vi "Main.vi"() -> ()   [LabVIEW 2016]
panel:
  in  "stop":bool
  in  "Tab Control":enum32{"Navigation", "Interface", "About"}(tab)
  in  "Reference Auto Update 3":bool=TRUE caption="Auto Update"
  out "move out":bool=TRUE caption="Move"
  in  "Positioner 2":u16(ring)=15 caption="Positioner" items=["ECGp5050", "ECGt5050", "ECR3030", "ECR4040", "ECR5050", "ECSx3030", "ECSx3040", "ECSx3050", "ECSx3060", "ECSx3070", "ECSx3080", "ECSx5050", "ECSxy5050", "ECSz3030", "ECSz5050", "EOP1", "EOP2"]
  out "in target range3":bool
  in  "auto Reset 1":bool=TRUE caption="Auto Reset"
  in  "Target Range 3":u32 caption="Target Range"
  in  "Reset Error 2":bool
  in  "Reset Error 3":bool
  out "Error 3":bool caption="Error"
  out "Error Message 3":string
  out "actor type 2":u16(ring) caption="Status" items=["linear positioner"=0, "rotator"=1, "goniometer"=2, "< error >"=9]
  out "actor type":u16(ring) caption="Status" items=["linear positioner"=0, "rotator"=1, "goniometer"=2, "< error >"=9]
  out "EotLeftDetected3":bool caption="Status Eot BWD"
  out "EotrightDetected3":bool caption="Status Eot FWD"
  in  "EoT 3":bool=TRUE caption="Stop on EoT"
  out "EotLeftDetected2":bool caption="Status Eot BWD"
  out "EotrightDetected2":bool caption="Status Eot FWD"
  in  "EoT 2":bool=TRUE caption="Stop on EoT"
  in  "Move 3":bool
  out "MoveSignal 3":bool caption="Positioner Connected/Moving"
  out "MoveSignal":bool caption="Positioner Connected/Moving"
  out "ReferenceSignal":bool=TRUE
  in  "Axis 3":bool caption="Closed Loop Funktions"
  in  "Axis 2":bool caption="Closed Loop Funktions"
  in  "Target Position 3":i32 caption="Target Position [µm]"
  in  "Target Position 1":i32 caption="Target position [µm]"
  in  "Number of steps 3":i32=1 caption="Number of Steps"
  in  "Number of steps 2":i32=1 caption="Number of Steps"
  in  "Output 2":bool caption="Axis 2"
  in  "Move 2":bool
  in  "Move":bool
  out "ReferenceSignal 3":bool
  out "Reference 3":dbl caption="Reference position [nm]" format="%#_6f"
  in  "Output":bool=TRUE caption="Axis 1"
  out "Output Satus 3":bool caption="Output Status"
  in  "Reference Auto Update 2":bool=TRUE caption="Auto Update"
  out "Error Message":string
  out "Error":bool
  in  "Output 3":bool caption="Axis 3"
  in  "auto Reset 3":bool=TRUE caption="Auto Reset"
  out "Output Status 1":bool=TRUE caption="Output Status"
  out "Position 3":dbl caption="Position [nm]" format="%#_6f"
  out "Output Status 2":bool caption="Output Status"
  in  "amplitude [V] 3":dbl=45.001 caption="Amplitude [V]" format="%#.3f"
  in  "frequency [Hz] 3":dbl=997.363 caption="Frequency [Hz]" format="%#.3f"
  out "Error 2":bool caption="Error"
  out "actor type 3":u16(ring) caption="Status" items=["linear positioner"=0, "rotator"=1, "goniometer"=2, "< error >"=9]
  out "Error Message 2":string
  out "Connected 3":bool caption="Connected"
  in  "Single Step Left 3":bool caption="Open Loop Funktions"
  in  "Positioner 3":u16(ring)=15 caption="Positioner" items=["ECGp5050", "ECGt5050", "ECR3030", "ECR4040", "ECR5050", "ECSx3030", "ECSx3040", "ECSx3050", "ECSx3060", "ECSx3070", "ECSx3080", "ECSx5050", "ECSxy5050", "ECSz3030", "ECSz5050", "EOP1", "EOP2"]
  in  "Endless Left 3":bool caption="Continuous Backward"
  in  "Continuous Forward":bool
  in  "Single Step Right 3":bool caption="Step(s)"
  in  "Fixed DC 3":i32 caption="DC Level [mV]"
  out "move out 3":bool=TRUE caption="Move"
  out "Position 2":dbl caption="Position [nm]" format="%#_6f"
  in  "amplitude [V] 2":dbl=45.001 caption="Amplitude [V]" format="%#.3f"
  in  "Amplitude [V]":dbl=45.001 format="%#.3f"
  in  "frequency [Hz] 2":dbl=997.363 caption="Frequency [Hz]" format="%#.3f"
  in  "Frequency [Hz]":dbl=1998.531 format="%#.3f"
  out "Connected 2":bool caption="Connected"
  in  "Single Step Left":bool caption="Open Loop Funktions"
  in  "Single Step Left 2":bool caption="Open Loop Funktions"
  in  "Single Step Right 2":bool caption="Step(s)"
  in  "Number of steps 1":i32=1 caption="Number of Steps"
  out "ReferenceSignal 2":bool
  in  "Single Step Right":bool caption="Step(s)"
  in  "Endless Left":bool caption="Continuous Backward"
  in  "Continuous Forward":bool
  in  "Endless Left 2":bool caption="Continuous Backward"
  out "EotLeftDetected1":bool caption="Status Eot BWD"
  out "EotrightDetected1":bool caption="Status Eot FWD"
  in  "EoT 1":bool caption="Stop on EoT"
  in  "Target position 2":i32 caption="Target Position [µm]"
  out "in target range2":bool
  in  "Continuous Forward":bool
  out "Reference 2":dbl caption="Reference position [nm]" format="%#_6f"
  in  "Fixed DC 2":i32 caption="DC Level [mV]"
  out "MoveSignal 2":bool caption="Positioner Connected/Moving"
  out "in target range1":bool
  in  "Target Range 2":u32 caption="Target Range [nm]"
  in  "Target Range 1":u32 caption="Target Range"
  out "Reference":dbl=-7597148.0 caption="Reference position [nm]" format="%#_6f"
  in  "auto Reset 2":bool=TRUE caption="Auto Reset"
  out "Position":dbl=14701.126 caption="Position [nm]" format="%#_6f"
  in  "Axis 1":bool caption="Closed Loop Funktions"
  in  "Fixed DC 1":i32 caption="DC Level [mV]"
  out "move out 2":bool=TRUE caption="Move"
  in  "Reset Error":bool
  out "Connected":bool=TRUE
  in  "Positioner":u16(ring)=15 items=["ECGp5050", "ECGt5050", "ECR3030", "ECR4040", "ECR5050", "ECSx3030", "ECSx3040", "ECSx3050", "ECSx3060", "ECSx3070", "ECSx3080", "ECSx5050", "ECSxy5050", "ECSz3030", "ECSz5050", "EOP1", "EOP2"]
  in  "Reference Auto Update 1":bool=TRUE caption="Auto Update"
  out "Error 4":bool caption="Error"
  out "Error Message 4":string
  in  "Mode Input 1":u16(ring) caption="Mode" items=["Trigger (LVDS)"=11, "Trigger (LVTTL)"=10, "Stepper (LVDS)"=9, "Stepper (LVTTL)"=8, "AquadB (LVDS)"=1, "AquadB (LVTTL)"=0, "OFF"=15]
  in  "Loop Mode 1":u16(ring) caption="Loop mode" items=["closed-loop"=1, "open-loop"=0]
  in  "Steps per pulse 1":i32 caption="Steps per pulse [Steps]"
  in  "Change per pulse 1":i32 caption="Change per pulse [u°/nm]"
  out "RT in move Signal 1":bool=TRUE caption="move"
  in  "RT in move 1":bool=TRUE caption="Move"
  in  "AquadB in res 1":i32 caption="AquadB Resolution [nm]"
  in  "AquadB out 1":bool caption="AquadB enable"
  in  "AqaudB clock 1":i32 caption="AquadB Clock [ns]"
  in  "AquadB Resolution 1":i32 caption="AquadB Resolution [nm]"
  in  "Reset Error 4":bool
  out "Error 5":bool caption="Error"
  out "Error Message 5":string
  in  "Mode Input 2":u16(ring) caption="Mode" items=["Trigger (LVDS)"=11, "Trigger (LVTTL)"=10, "Stepper (LVDS)"=9, "Stepper (LVTTL)"=8, "AquadB (LVDS)"=1, "AquadB (LVTTL)"=0, "OFF"=15]
  in  "Loop Mode 2":u16(ring) caption="Loop mode" items=["closed-loop"=1, "open-loop"=0]
  in  "Steps per pulse 2":i32 caption="Steps per pulse [Steps]"
  in  "Change per pulse 2":i32 caption="Change per pulse  [u°/nm]"
  out "RT in move Signal 2":bool=TRUE caption="move"
  in  "RT in move 2":bool=TRUE caption="Move"
  in  "AquadB in res 2":i32 caption="AquadB Resolution [nm]"
  in  "AquadB out 2":bool caption="AquadB enable"
  in  "AqaudB clock 2":i32 caption="AquadB Clock [ns]"
  in  "AquadB Resolution 2":i32 caption="AquadB Resolution [nm]"
  in  "Reset Error 5":bool
  out "Error 6":bool caption="Error"
  out "Error Message 6":string
  in  "Mode Input 3":u16(ring) caption="Mode" items=["Trigger (LVDS)"=11, "Trigger (LVTTL)"=10, "Stepper (LVDS)"=9, "Stepper (LVTTL)"=8, "AquadB (LVDS)"=1, "AquadB (LVTTL)"=0, "OFF"=15]
  in  "Loop Mode 3":u16(ring) caption="Loop mode" items=["closed-loop"=1, "open-loop"=0]
  in  "Steps per pulse 3":i32 caption="Steps per pulse [Steps]"
  in  "Change per pulse 3":i32 caption="Change per pulse  [u°/nm]"
  out "RT in move Signal 3":bool=TRUE caption="move"
  in  "RT in move 3":bool=TRUE caption="Move"
  in  "AquadB in res 3":i32 caption="AquadB Resolution [nm]"
  in  "Output Mode":u16(ring) caption="Mode" items=["AquadB (LVTTL)", "AquadB (LVDS)"]
  in  "AquadB out 3":bool caption="AquadB enable"
  in  "AqaudB clock 3":i32 caption="AquadB Clock [ns]"
  in  "AquadB Resolution 3":i32 caption="AquadB Resolution [nm]"
  in  "Reset Error 6":bool
  in  "Reboot":bool
  in  "Factory Reset":bool
  in  "Reset Error 8":bool
  out "Error Message 7":string
  in  "Lock password":string
  in  "name":string="Test" caption="Device Name"
  in  "Access Password":string
  out "Error 7":bool caption="Error"
  out "locked":bool
  out "authorized":bool
  in  "Unlock":bool=TRUE
  out "Name":string caption="Device Name"
  out "Device type":string="AMC100/NUM"
  out "Sn":string caption="Serial Number"
  out "ip":string="192.168.1.1" caption="IP Adress"
  out "Firmware Version":string
  out "FPGA Version":string
  out "Mac Adress":string
  # "Real Time Input"
  # "Real Time Output"
  # "Global Parameters"
  # "Axis 1"
  # "Axis 1"
  # "Axis 2"
  # "Axis 2"
  # "Axis 3"
  # "Axis 3"
  # "Device Info"
  # "Device Access"
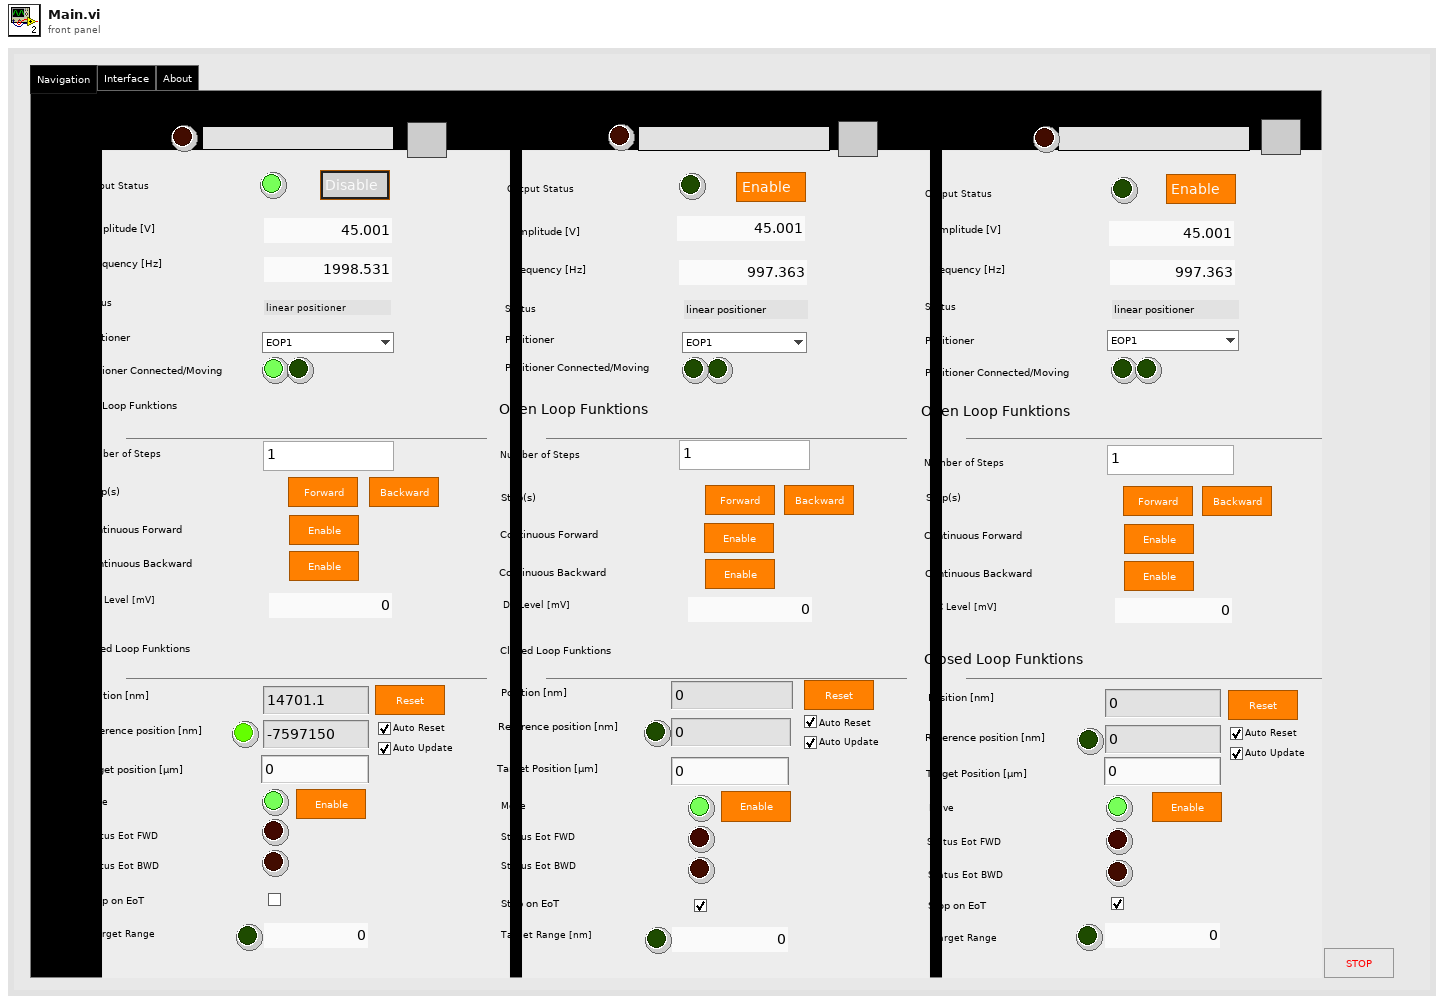
[diagram p1: front panel]
types:
  T1 = enum8{"Enabled", "Disabled", "Disabled and Grayed Out"}
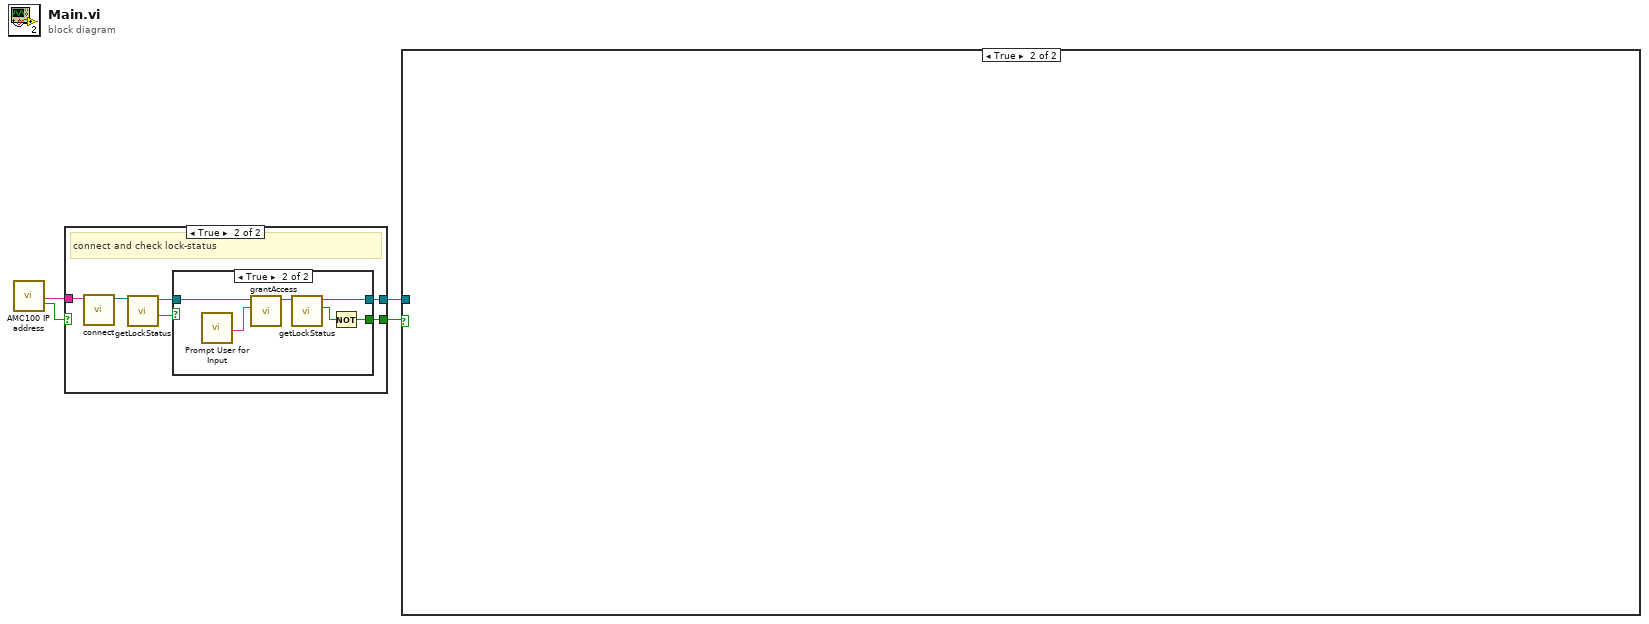
[diagram p0: block diagram]
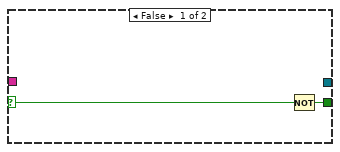
[diagram p2: hidden frame]
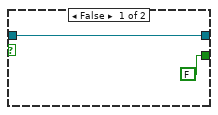
[diagram p3: hidden frame]
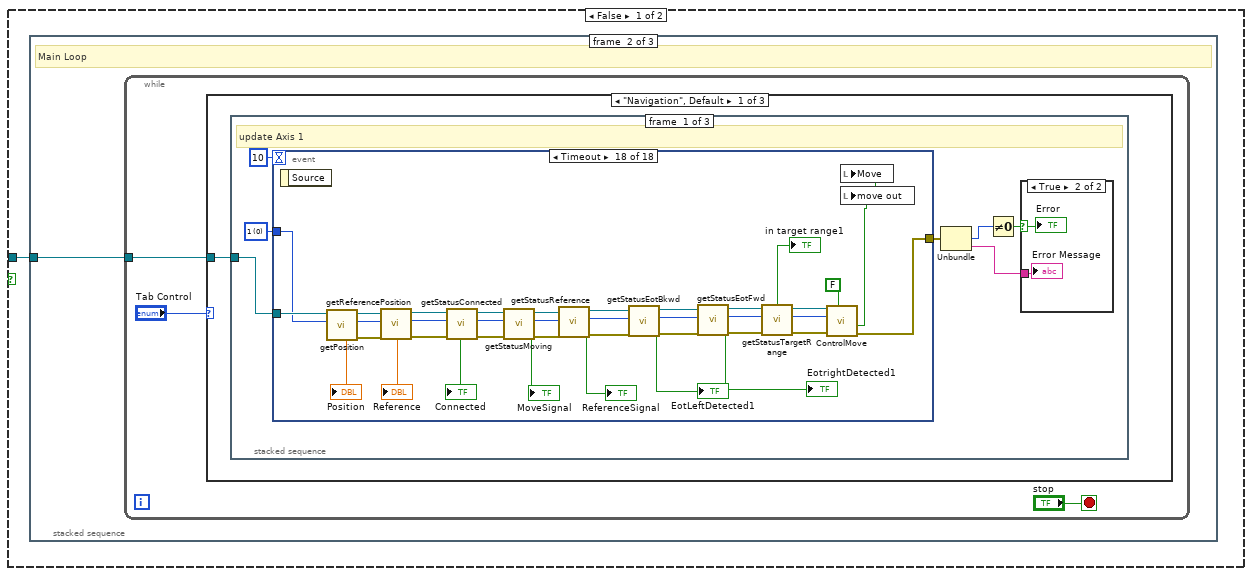
[diagram p4: hidden frame]
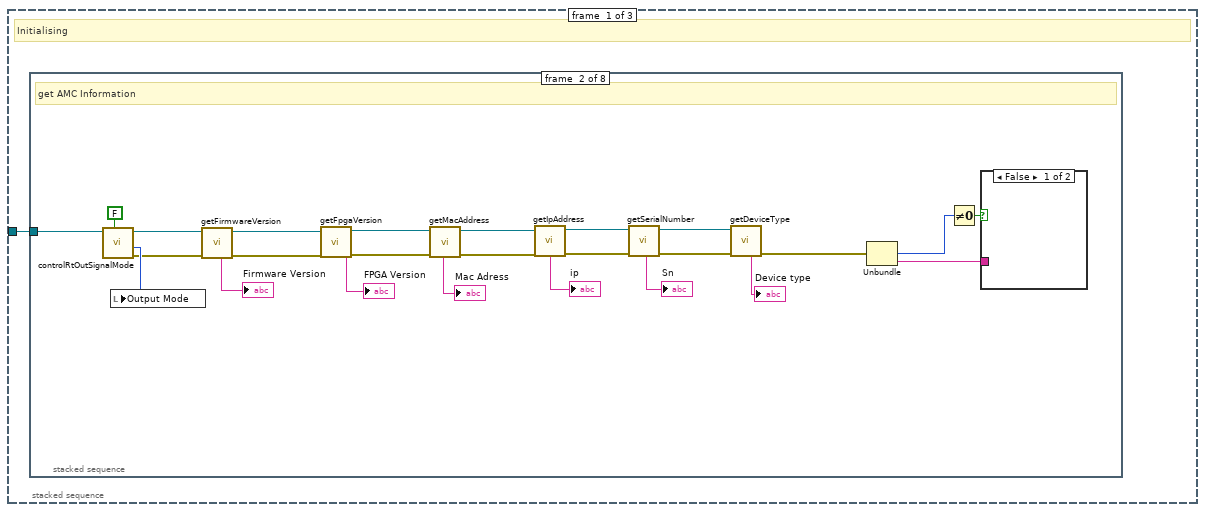
[diagram p5: hidden frame]
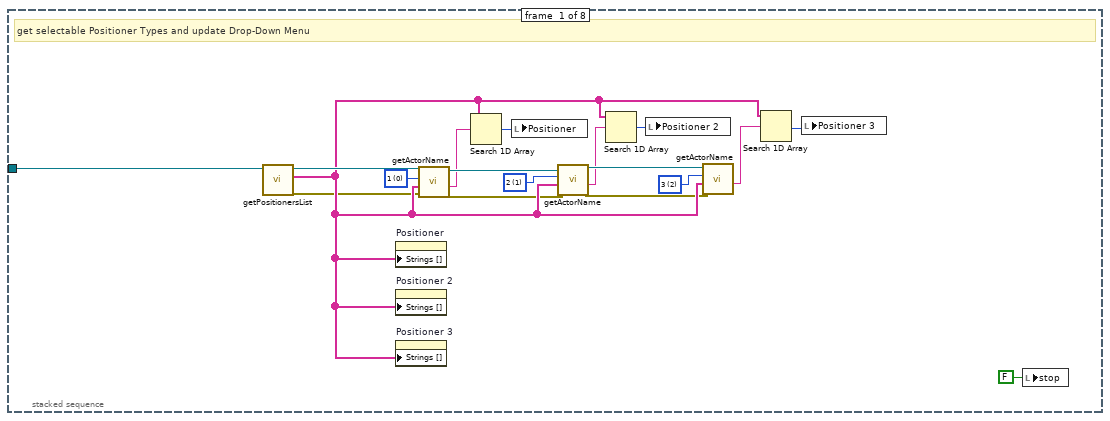
[diagram p6: hidden frame]
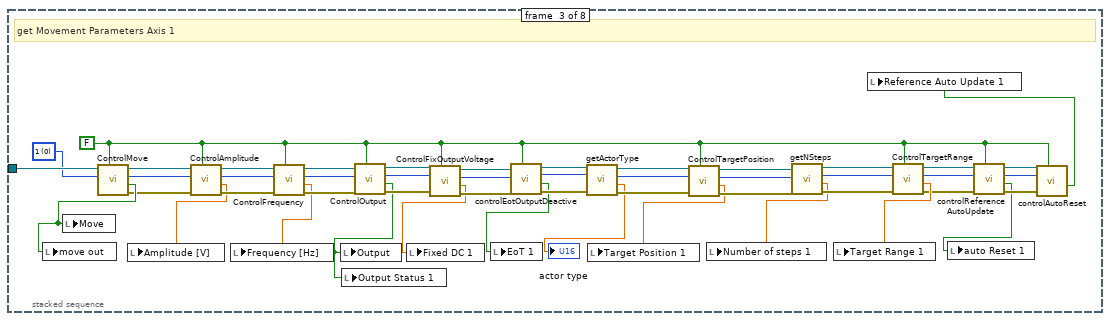
[diagram p8: hidden frame]
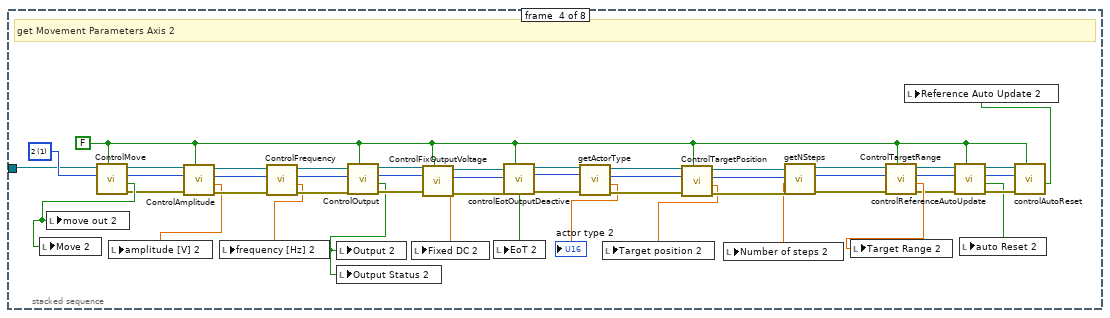
[diagram p9: hidden frame]
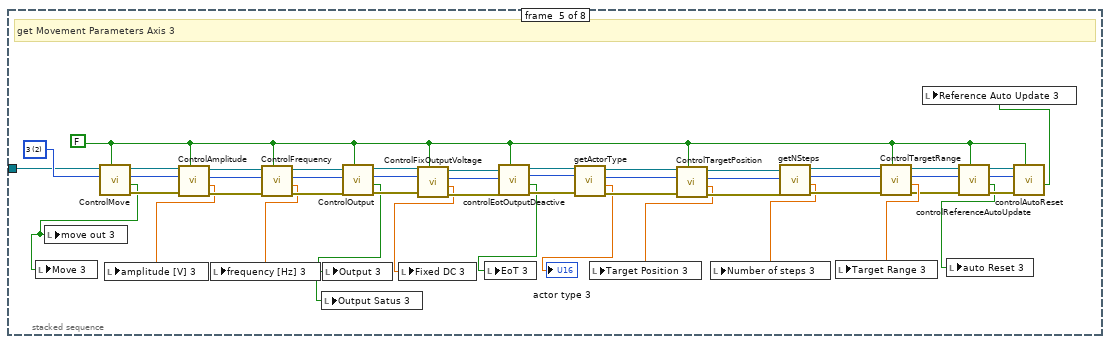
[diagram p10: hidden frame]
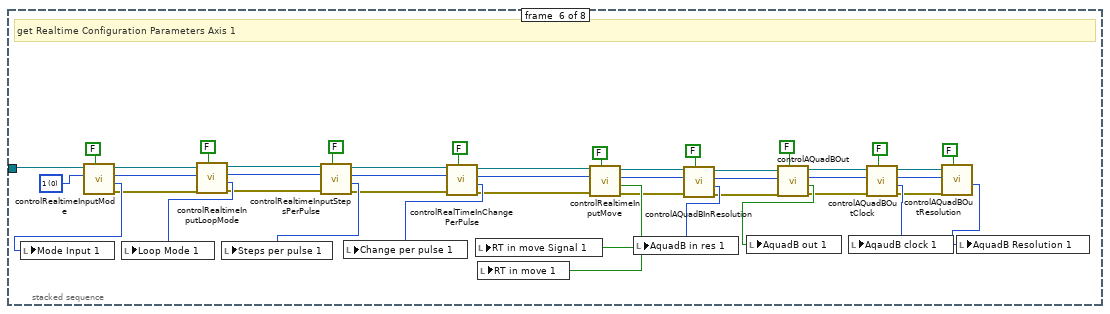
[diagram p11: hidden frame]
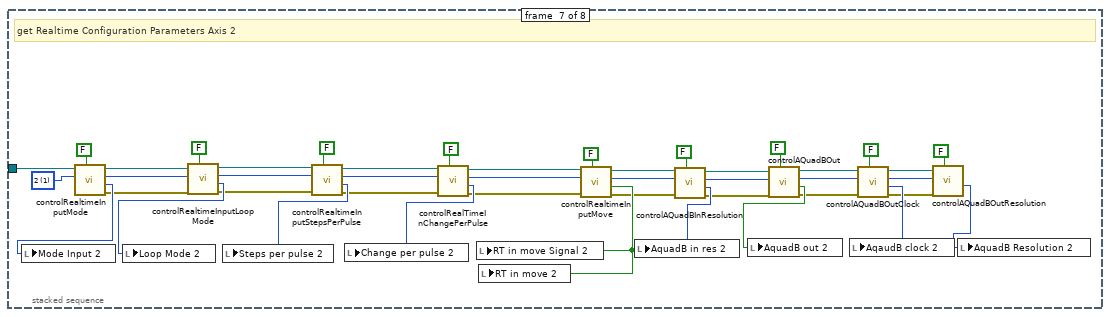
[diagram p12: hidden frame]
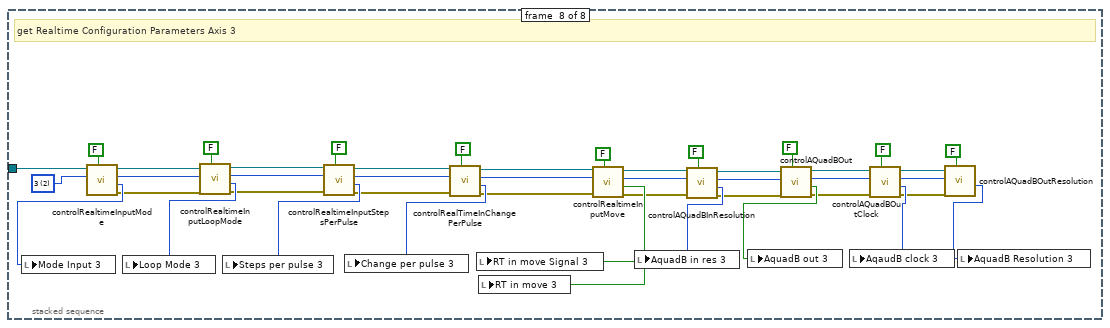
[diagram p13: hidden frame]
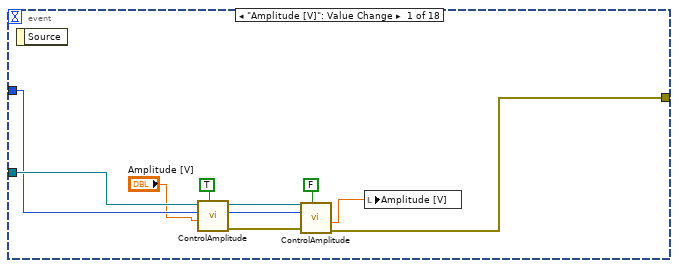
[diagram p15: hidden frame]
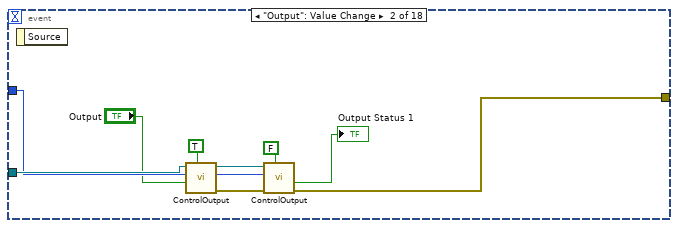
[diagram p16: hidden frame]
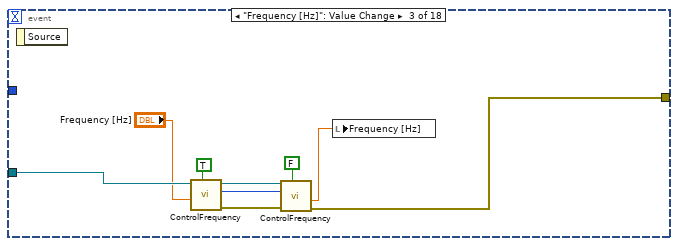
[diagram p17: hidden frame]
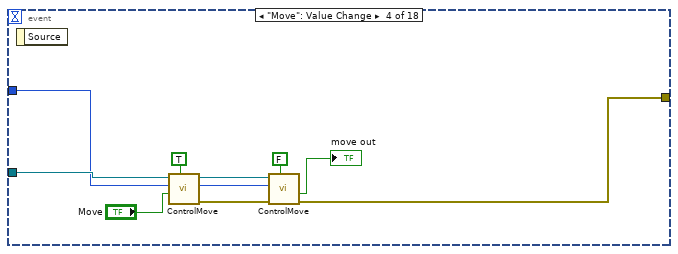
[diagram p18: hidden frame]
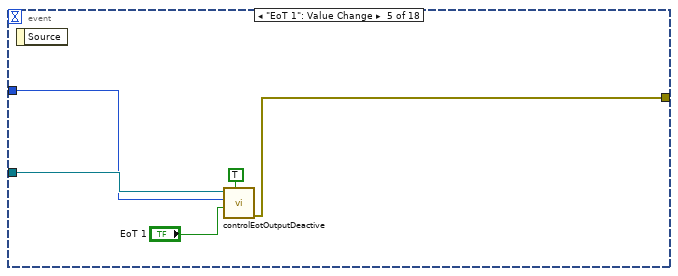
[diagram p19: hidden frame]
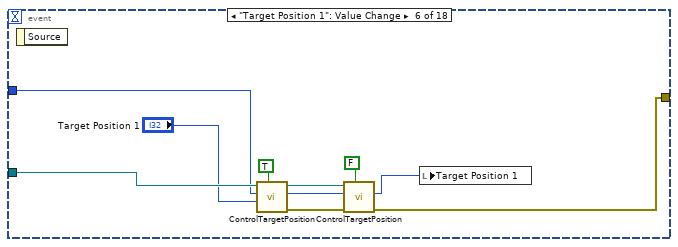
[diagram p20: hidden frame]
diagram:
  n1 = call "AMC100 IP address"() -> ("IP address"=w1:string, "OK"=w2:bool)  [unwired: 17 in, 1 out]
  n2 = case shown="True" w2 {
    selector: w2 -> [w5 _]
    tunnel: [w6 w12] -> w4
    tunnel: [_ w11] -> w3
    tunnel: w1 -> [_ w7]
    frame False {
      n3 = Not(x=w5) -> (.not. x?=w6:bool)
    }
    frame True {
      # "connect and check lock-status"
      n4 = call "connect.vi"("deviceAddress"=w7) -> ("connection ID"=w10:refnum<k5>)  [unwired: 5 in, 1 out]
      n5 = call "getLockStatus.vi"("connection ID in"=w10) -> ("locked"=w8:bool, "connection ID out"=w9:refnum<k5>)  [unwired: 7 in, 2 out]
      n6 = case shown="True" w8 {
        tunnel: w9 -> [w14 w20]
        tunnel: [w14 w17] -> w11
        tunnel: [FALSE w16] -> w12
        frame False {
        }
        frame True {
          n7 = call "Prompt User for Input"() -> ("password"=w19:string)  [unwired: 17 in, 2 out]
          n8 = call "grantAccess.vi"("password"=w19, "connection ID"=w20) -> ("connection ID"=w18:refnum<k5>)  [unwired: 8 in, 1 out]
          n9 = call "getLockStatus.vi"("connection ID in"=w18) -> ("authorized"=w15:bool, "connection ID out"=w17:refnum<k5>)  [unwired: 7 in, 2 out]
          n10 = Not(x=w15) -> (.not. x?=w16:bool)
        }
      }
    }
  }
  n11 = case shown="True" w4 {
    tunnel: w3 -> [w21 _]
    frame False {
      n12 = stacked-sequence {
        tunnel: w21 -> [w22 w342 w1332]
        frame #0 {
          # "Initialising"
          n13 = stacked-sequence {
            tunnel: w22 -> [w40 w44 w72 w120 w166 w253 w297 w341]
            frame #0 {
              w37 = u8 2 items=["1", "2", "3"] ("axis")
              w34 = u8 1 items=["1", "2", "3"] ("axis")
              w31 = u8 0 items=["1", "2", "3"] ("axis")
              # "get selectable Positioner Types and update Drop-Down Menu"
              n14 = call "getPositionersList.vi"("connection ID"=w40) -> ("error out"=w23:errorcluster, "Positioners List"=w26:string[], "connection ID"=w30:refnum<k5>)  [unwired: 8 in]
              n15 = property on="Positioner" class="Ring (strict)"("Strings []"=w26) -> ()  [unwired: 2 in, 2 out]
              n16 = property on="Positioner 2" class="Ring (strict)"("Strings []"=w26) -> ()  [unwired: 2 in, 2 out]
              n17 = property on="Positioner 3" class="Ring (strict)"("Strings []"=w26) -> ()  [unwired: 2 in, 2 out]
              n18 = call "getActorName.vi"("error in"=w23, "Actor Names"=w26, "axis in"=w31, "connection ID"=w30) -> ("error out"=w25:errorcluster, "ActorName out"=w32:string, "connection ID"=w33:refnum<k5>)  [unwired: 4 in, 1 out]
              n19 = Search 1D Array(1D array=w26, element=w32) -> (index of element=w27:i32)  [unwired: 1 in]
              n20 = local write "Positioner"(w27) -> ()
              n21 = call "getActorName.vi"("error in"=w25, "Actor Names"=w26, "axis in"=w34, "connection ID"=w33) -> ("error out"=w24:errorcluster, "ActorName out"=w35:string, "connection ID"=w36:refnum<k5>)  [unwired: 4 in, 1 out]
              n22 = Search 1D Array(1D array=w26, element=w35) -> (index of element=w28:i32)  [unwired: 1 in]
              n23 = local write "Positioner 2"(w28) -> ()
              n24 = call "getActorName.vi"("error in"=w24, "Actor Names"=w26, "axis in"=w37, "connection ID"=w36) -> ("ActorName out"=w38:string)  [unwired: 4 in, 3 out]
              n25 = Search 1D Array(1D array=w26, element=w38) -> (index of element=w29:i32)  [unwired: 1 in]
              n26 = local write "Positioner 3"(w29) -> ()
              n27 = local write "stop"(FALSE ("stop")) -> ()
            }
            frame #1 {
              # "get AMC Information"
              n28 = call "controlRtOutSignalMode.vi"("Set"=FALSE, "connection ID"=w44) -> ("error out"=w42:errorcluster, "RT out Mode out"=w45:i32, "connection ID"=w43:refnum<k5>)  [unwired: 7 in]
              n29 = local write "Output Mode"(w45) -> ()
              n30 = call "getFirmwareVersion.vi"("error in"=w42, "connection ID"=w43) -> ("error out"=w51:errorcluster, "Firmware Version out"=→"Firmware Version":string, "connection ID"=w61:refnum<k5>)  [unwired: 7 in]
              n31 = call "getFpgaVersion.vi"("error in"=w51, "connection ID"=w61) -> ("error out"=w50:errorcluster, "FPGA out"=→"FPGA Version":string, "connection ID"=w59:refnum<k5>)  [unwired: 7 in]
              n32 = call "getMacAddress.vi"("error in"=w50, "connection ID"=w59) -> ("error out"=w49:errorcluster, "Mac Adress out"=→"Mac Adress":string, "connection ID"=w56:refnum<k5>)  [unwired: 7 in]
              n33 = call "getIpAddress.vi"("error in"=w49, "connection ID"=w56) -> ("error out"=w48:errorcluster, "IP out"=→"ip":string, "connection ID"=w55:refnum<k5>)  [unwired: 7 in]
              n34 = call "getSerialNumber.vi"("error in"=w48, "connection ID"=w55) -> ("error out"=w47:errorcluster, "sn out"=→"Sn":string, "connection ID"=w53:refnum<k5>)  [unwired: 7 in]
              n35 = call "getDeviceType.vi"("error in"=w47, "connection ID"=w53) -> ("error out"=w41:errorcluster, "Device Type out"=→"Device type":string)  [unwired: 7 in, 1 out]
              n36 = Unbundle(w41) -> ("code"=w64:i32, "source"=w65:string)  [unwired: 1 out]
              n37 = Not Equal To 0?(x=w64) -> (x != 0?=w63:bool)
              n38 = case shown="False" w63 {
                tunnel: w65 -> [_ _]
                frame False {
                }
                frame True {
                }
              }
            }
            frame #2 {
              w70 = u8 0 items=["1", "2", "3"] ("axis")
              w73 = FALSE ("set")
              # "get Movement Parameters Axis 1"
              n39 = call "ControlMove.vi"("Set"=w73, "axis in"=w70, "connection ID"=w72) -> ("error out"=w67:errorcluster, "controll move out"=w68:bool, "axis out"=w69:u8, "connection ID"=w71:refnum<k5>)  [unwired: 5 in]
              n40 = local write "move out"(w68) -> ()
              n41 = local write "Move"(w68) -> ()
              n42 = call "ControlAmplitude.vi"("Set"=w73, "error in"=w67, "axis in"=w69, "connection ID"=w71) -> ("error out"=w111:errorcluster, "amplitude [V] out"=w89:dbl, "axis out"=w113:u8, "connection ID"=w112:refnum<k5>)  [unwired: 4 in]
              n43 = local write "Amplitude [V]"(w89) -> ()
              n44 = call "ControlFrequency.vi"("Set"=w73, "error in"=w111, "axis in"=w113, "connection ID"=w112) -> ("error out"=w108:errorcluster, "Frequency [Hz] out"=w88:dbl, "axis out"=w109:u8, "connection ID"=w110:refnum<k5>)  [unwired: 4 in]
              n45 = local write "Frequency [Hz]"(w88) -> ()
              n46 = call "ControlOutput.vi"("Set"=w73, "error in"=w108, "axis in"=w109, "connection ID"=w110) -> ("error out"=w105:errorcluster, "enable output out"=w66:bool, "axis out"=w106:u8, "connection ID"=w107:refnum<k5>)  [unwired: 4 in]
              n47 = local write "Output"(w66) -> ()
              n48 = local write "Output Status 1"(w66) -> ()
              n49 = call "ControlFixOutputVoltage.vi"("Set"=w73, "error in"=w105, "axis in"=w106, "connection ID"=w107) -> ("error out"=w102:errorcluster, "Fixed Output Voltage out"=w87:dbl, "axis out"=w103:u8, "connection ID"=w104:refnum<k5>)  [unwired: 4 in]
              n50 = local write "Fixed DC 1"(w87) -> ()
              n51 = call "controlEotOutputDeactive.vi"("Set"=w73, "error in"=w102, "axis in"=w103, "connection ID"=w104) -> ("error out"=w99:errorcluster, "enable EOT out"=w86:bool, "axis out"=w100:u8, "connection ID"=w101:refnum<k5>)  [unwired: 4 in]
              n52 = local write "EoT 1"(w86) -> ()
              n53 = call "getActorType.vi"("error in"=w99, "axis in"=w100, "connection ID"=w101) -> ("error out"=w96:errorcluster, "Actor Type"=→"actor type":dbl, "axis out"=w97:u8, "connection ID"=w98:refnum<k5>)  [unwired: 5 in]
              n54 = call "ControlTargetPosition.vi"("Set"=w73, "error in"=w96, "axis in"=w97, "connection ID"=w98) -> ("error out"=w93:errorcluster, "Target Position out"=w84:dbl, "axis out"=w94:u8, "connection ID"=w95:refnum<k5>)  [unwired: 4 in]
              n55 = local write "Target Position 1"(w84) -> ()
              n56 = call "getNSteps.vi"("error in"=w93, "axis in"=w94, "connection ID"=w95) -> ("error out"=w90:errorcluster, "setnSteps out"=w83:dbl, "axis out"=w91:u8, "connection ID"=w92:refnum<k5>)  [unwired: 5 in]
              n57 = local write "Number of steps 1"(w83) -> ()
              n58 = call "ControlTargetRange.vi"("Set"=w73, "error in"=w90, "axis in"=w91, "connection ID"=w92) -> ("error out"=w79:errorcluster, "Target Range out"=w82:dbl, "axis out"=w80:u8, "connection ID"=w81:refnum<k5>)  [unwired: 4 in]
              n59 = local write "Target Range 1"(w82) -> ()
              n60 = call "controlReferenceAutoUpdate.vi"("Set"=w73, "error in"=w79, "axis in"=w80, "connection ID"=w81) -> ("error out"=w76:errorcluster, "ref auto up out"=w75:bool, "axis out"=w77:u8, "connection ID"=w78:refnum<k5>)  [unwired: 4 in]
              n61 = local write "auto Reset 1"(w75) -> ()
              n62 = call "controlAutoReset.vi"("Set"=w73, "error in"=w76, "axis in"=w77, "connection ID"=w78) -> ("auto reset out"=w74:bool)  [unwired: 4 in, 3 out]
              n63 = local write "Reference Auto Update 1"(w74) -> ()
            }
            frame #3 {
              w121 = u8 1 items=["1", "2", "3"] ("axis")
              w114 = FALSE ("set")
              # "get Movement Parameters Axis 2"
              n64 = call "ControlMove.vi"("Set"=w114, "axis in"=w121, "connection ID"=w120) -> ("error out"=w116:errorcluster, "controll move out"=w119:bool, "axis out"=w117:u8, "connection ID"=w118:refnum<k5>)  [unwired: 5 in]
              n65 = local write "Move 2"(w119) -> ()
              n66 = local write "move out 2"(w119) -> ()
              n67 = call "ControlAmplitude.vi"("Set"=w114, "error in"=w116, "axis in"=w117, "connection ID"=w118) -> ("error out"=w159:errorcluster, "amplitude [V] out"=w137:dbl, "axis out"=w161:u8, "connection ID"=w160:refnum<k5>)  [unwired: 4 in]
              n68 = local write "amplitude [V] 2"(w137) -> ()
              n69 = call "ControlFrequency.vi"("error in"=w159, "axis in"=w161, "connection ID"=w160) -> ("error out"=w156:errorcluster, "Frequency [Hz] out"=w136:dbl, "axis out"=w157:u8, "connection ID"=w158:refnum<k5>)  [unwired: 5 in]
              n70 = local write "frequency [Hz] 2"(w136) -> ()
              n71 = call "ControlOutput.vi"("Set"=w114, "error in"=w156, "axis in"=w157, "connection ID"=w158) -> ("error out"=w153:errorcluster, "enable output out"=w115:bool, "axis out"=w154:u8, "connection ID"=w155:refnum<k5>)  [unwired: 4 in]
              n72 = local write "Output 2"(w115) -> ()
              n73 = local write "Output Status 2"(w115) -> ()
              n74 = call "ControlFixOutputVoltage.vi"("Set"=w114, "error in"=w153, "axis in"=w154, "connection ID"=w155) -> ("error out"=w150:errorcluster, "Fixed Output Voltage out"=w135:dbl, "axis out"=w151:u8, "connection ID"=w152:refnum<k5>)  [unwired: 4 in]
              n75 = local write "Fixed DC 2"(w135) -> ()
              n76 = call "controlEotOutputDeactive.vi"("Set"=w114, "error in"=w150, "axis in"=w151, "connection ID"=w152) -> ("error out"=w147:errorcluster, "enable EOT out"=w134:bool, "axis out"=w148:u8, "connection ID"=w149:refnum<k5>)  [unwired: 4 in]
              n77 = local write "EoT 2"(w134) -> ()
              n78 = call "getActorType.vi"("error in"=w147, "axis in"=w148, "connection ID"=w149) -> ("error out"=w144:errorcluster, "Actor Type"=→"actor type 2":dbl, "axis out"=w145:u8, "connection ID"=w146:refnum<k5>)  [unwired: 5 in]
              n79 = call "ControlTargetPosition.vi"("Set"=w114, "error in"=w144, "axis in"=w145, "connection ID"=w146) -> ("error out"=w141:errorcluster, "Target Position out"=w132:dbl, "axis out"=w142:u8, "connection ID"=w143:refnum<k5>)  [unwired: 4 in]
              n80 = local write "Target position 2"(w132) -> ()
              n81 = call "getNSteps.vi"("error in"=w141, "axis in"=w142, "connection ID"=w143) -> ("error out"=w138:errorcluster, "setnSteps out"=w131:dbl, "axis out"=w139:u8, "connection ID"=w140:refnum<k5>)  [unwired: 5 in]
              n82 = local write "Number of steps 2"(w131) -> ()
              n83 = call "ControlTargetRange.vi"("Set"=w114, "error in"=w138, "axis in"=w139, "connection ID"=w140) -> ("error out"=w125:errorcluster, "Target Range out"=w130:dbl, "axis out"=w127:u8, "connection ID"=w129:refnum<k5>)  [unwired: 4 in]
              n84 = local write "Target Range 2"(w130) -> ()
              n85 = call "controlReferenceAutoUpdate.vi"("Set"=w114, "error in"=w125, "axis in"=w127, "connection ID"=w129) -> ("error out"=w124:errorcluster, "ref auto up out"=w123:bool, "axis out"=w126:u8, "connection ID"=w128:refnum<k5>)  [unwired: 4 in]
              n86 = local write "auto Reset 2"(w123) -> ()
              n87 = call "controlAutoReset.vi"("Set"=w114, "error in"=w124, "axis in"=w126, "connection ID"=w128) -> ("auto reset out"=w122:bool)  [unwired: 4 in, 3 out]
              n88 = local write "Reference Auto Update 2"(w122) -> ()
            }
            frame #4 {
              w167 = u8 2 items=["1", "2", "3"] ("axis")
              w165 = FALSE ("set")
              # "get Movement Parameters Axis 3"
              n89 = call "ControlMove.vi"("Set"=w165, "axis in"=w167, "connection ID"=w166) -> ("error out"=w164:errorcluster, "controll move out"=w163:bool, "axis out"=w168:u8, "connection ID"=w169:refnum<k5>)  [unwired: 5 in]
              n90 = local write "Move 3"(w163) -> ()
              n91 = local write "move out 3"(w163) -> ()
              n92 = call "ControlAmplitude.vi"("Set"=w165, "error in"=w164, "axis in"=w168, "connection ID"=w169) -> ("error out"=w207:errorcluster, "amplitude [V] out"=w185:dbl, "axis out"=w209:u8, "connection ID"=w208:refnum<k5>)  [unwired: 4 in]
              n93 = local write "amplitude [V] 3"(w185) -> ()
              n94 = call "ControlFrequency.vi"("Set"=w165, "error in"=w207, "axis in"=w209, "connection ID"=w208) -> ("error out"=w204:errorcluster, "Frequency [Hz] out"=w184:dbl, "axis out"=w205:u8, "connection ID"=w206:refnum<k5>)  [unwired: 4 in]
              n95 = local write "frequency [Hz] 3"(w184) -> ()
              n96 = call "ControlOutput.vi"("Set"=w165, "error in"=w204, "axis in"=w205, "connection ID"=w206) -> ("error out"=w201:errorcluster, "enable output out"=w162:bool, "axis out"=w202:u8, "connection ID"=w203:refnum<k5>)  [unwired: 4 in]
              n97 = local write "Output Satus 3"(w162) -> ()
              n98 = local write "Output 3"(w162) -> ()
              n99 = call "ControlFixOutputVoltage.vi"("Set"=w165, "error in"=w201, "axis in"=w202, "connection ID"=w203) -> ("error out"=w198:errorcluster, "Fixed Output Voltage out"=w183:dbl, "axis out"=w199:u8, "connection ID"=w200:refnum<k5>)  [unwired: 4 in]
              n100 = local write "Fixed DC 3"(w183) -> ()
              n101 = call "controlEotOutputDeactive.vi"("Set"=w165, "error in"=w198, "axis in"=w199, "connection ID"=w200) -> ("error out"=w195:errorcluster, "enable EOT out"=w182:bool, "axis out"=w196:u8, "connection ID"=w197:refnum<k5>)  [unwired: 4 in]
              n102 = local write "EoT 3"(w182) -> ()
              n103 = call "getActorType.vi"("error in"=w195, "axis in"=w196, "connection ID"=w197) -> ("error out"=w192:errorcluster, "Actor Type"=→"actor type 3":dbl, "axis out"=w193:u8, "connection ID"=w194:refnum<k5>)  [unwired: 5 in]
              n104 = call "ControlTargetPosition.vi"("Set"=w165, "error in"=w192, "axis in"=w193, "connection ID"=w194) -> ("error out"=w189:errorcluster, "Target Position out"=w181:dbl, "axis out"=w190:u8, "connection ID"=w191:refnum<k5>)  [unwired: 4 in]
              n105 = local write "Target Position 3"(w181) -> ()
              n106 = call "getNSteps.vi"("error in"=w189, "axis in"=w190, "connection ID"=w191) -> ("error out"=w186:errorcluster, "setnSteps out"=w180:dbl, "axis out"=w187:u8, "connection ID"=w188:refnum<k5>)  [unwired: 5 in]
              n107 = local write "Number of steps 3"(w180) -> ()
              n108 = call "ControlTargetRange.vi"("Set"=w165, "error in"=w186, "axis in"=w187, "connection ID"=w188) -> ("error out"=w172:errorcluster, "Target Range out"=w179:dbl, "axis out"=w173:u8, "connection ID"=w174:refnum<k5>)  [unwired: 4 in]
              n109 = local write "Target Range 3"(w179) -> ()
              n110 = call "controlReferenceAutoUpdate.vi"("Set"=w165, "error in"=w172, "axis in"=w173, "connection ID"=w174) -> ("error out"=w175:errorcluster, "ref auto up out"=w171:bool, "axis out"=w176:u8, "connection ID"=w177:refnum<k5>)  [unwired: 4 in]
              n111 = local write "auto Reset 3"(w171) -> ()
              n112 = call "controlAutoReset.vi"("Set"=w165, "error in"=w175, "axis in"=w176, "connection ID"=w177) -> ("auto reset out"=w170:bool)  [unwired: 4 in, 3 out]
              n113 = local write "Reference Auto Update 3"(w170) -> ()
            }
            frame #5 {
              w211 = u8 0 items=["1", "2", "3"] ("axis")
              # "get Realtime Configuration Parameters Axis 1"
              n114 = call "controlRealtimeInputMode.vi"("Set"=FALSE, "axis in"=w211, "connection ID"=w253) -> ("error out"=w228:errorcluster, "RT Mode out"=w252:i32, "axis out"=w220:u8, "connection ID"=w212:refnum<k5>)  [unwired: 5 in]
              n115 = local write "Mode Input 1"(w252) -> ()
              n116 = call "controlRealtimeInputLoopMode.vi"("Set"=FALSE, "error in"=w228, "axis in"=w220, "connection ID"=w212) -> ("error out"=w229:errorcluster, "RT Loop out"=w251:i32, "axis out"=w221:u8, "connection ID"=w213:refnum<k5>)  [unwired: 4 in]
              n117 = local write "Loop Mode 1"(w251) -> ()
              n118 = call "controlRealtimeInputStepsPerPulse.vi"("Set"=FALSE, "error in"=w229, "axis in"=w221, "connection ID"=w213) -> ("error out"=w230:errorcluster, "Steps out"=w250:i32, "axis out"=w222:u8, "connection ID"=w214:refnum<k5>)  [unwired: 4 in]
              n119 = local write "Steps per pulse 1"(w250) -> ()
              n120 = call "controlRealTimeInChangePerPulse.vi"("Set"=FALSE, "error in"=w230, "axis in"=w222, "connection ID"=w214) -> ("error out"=w231:errorcluster, "Change out"=w249:i32, "axis out"=w223:u8, "connection ID"=w215:refnum<k5>)  [unwired: 4 in]
              n121 = local write "Change per pulse 1"(w249) -> ()
              n122 = call "controlRealtimeInputMove.vi"("Set"=FALSE, "error in"=w231, "axis in"=w223, "connection ID"=w215) -> ("error out"=w232:errorcluster, "move out"=w248:bool, "axis out"=w224:u8, "connection ID"=w216:refnum<k5>)  [unwired: 4 in]
              n123 = local write "RT in move Signal 1"(w248) -> ()
              n124 = local write "RT in move 1"(w248) -> ()
              n125 = call "controlAQuadBInResolution.vi"("Set"=FALSE, "error in"=w232, "axis in"=w224, "connection ID"=w216) -> ("error out"=w233:errorcluster, "Resolution out"=w247:i32, "axis out"=w225:u8, "connection ID"=w217:refnum<k5>)  [unwired: 3 in]
              n126 = local write "AquadB in res 1"(w247) -> ()
              n127 = call "controlAQuadBOut.vi"("Set"=FALSE, "error in"=w233, "axis in"=w225, "connection ID"=w217) -> ("error out"=w234:errorcluster, "ABout out"=w246:bool, "axis out"=w226:u8, "connection ID"=w218:refnum<k5>)  [unwired: 4 in]
              n128 = local write "AquadB out 1"(w246) -> ()
              n129 = call "controlAQuadBOutClock.vi"("Set"=FALSE, "error in"=w234, "axis in"=w226, "connection ID"=w218) -> ("error out"=w235:errorcluster, "clock out"=w245:i32, "axis out"=w227:u8, "connection ID"=w219:refnum<k5>)  [unwired: 4 in]
              n130 = local write "AqaudB clock 1"(w245) -> ()
              n131 = call "controlAQuadBOutResolution.vi"("Set"=FALSE, "error in"=w235, "axis in"=w227, "connection ID"=w219) -> ("ABoutRes out"=w244:i32)  [unwired: 4 in, 3 out]
              n132 = local write "AquadB Resolution 1"(w244) -> ()
            }
            frame #6 {
              w255 = u8 1 items=["1", "2", "3"] ("axis")
              # "get Realtime Configuration Parameters Axis 2"
              n133 = call "controlRealtimeInputMode.vi"("Set"=FALSE, "axis in"=w255, "connection ID"=w297) -> ("error out"=w272:errorcluster, "RT Mode out"=w296:i32, "axis out"=w264:u8, "connection ID"=w256:refnum<k5>)  [unwired: 5 in]
              n134 = local write "Mode Input 2"(w296) -> ()
              n135 = call "controlRealtimeInputLoopMode.vi"("Set"=FALSE, "error in"=w272, "axis in"=w264, "connection ID"=w256) -> ("error out"=w273:errorcluster, "RT Loop out"=w295:i32, "axis out"=w265:u8, "connection ID"=w257:refnum<k5>)  [unwired: 4 in]
              n136 = local write "Loop Mode 2"(w295) -> ()
              n137 = call "controlRealtimeInputStepsPerPulse.vi"("Set"=FALSE, "error in"=w273, "axis in"=w265, "connection ID"=w257) -> ("error out"=w274:errorcluster, "Steps out"=w294:i32, "axis out"=w266:u8, "connection ID"=w258:refnum<k5>)  [unwired: 4 in]
              n138 = local write "Steps per pulse 2"(w294) -> ()
              n139 = call "controlRealTimeInChangePerPulse.vi"("Set"=FALSE, "error in"=w274, "axis in"=w266, "connection ID"=w258) -> ("error out"=w275:errorcluster, "Change out"=w293:i32, "axis out"=w267:u8, "connection ID"=w259:refnum<k5>)  [unwired: 4 in]
              n140 = local write "Change per pulse 2"(w293) -> ()
              n141 = call "controlRealtimeInputMove.vi"("Set"=FALSE, "error in"=w275, "axis in"=w267, "connection ID"=w259) -> ("error out"=w276:errorcluster, "move out"=w292:bool, "axis out"=w268:u8, "connection ID"=w260:refnum<k5>)  [unwired: 4 in]
              n142 = local write "RT in move Signal 2"(w292) -> ()
              n143 = local write "RT in move 2"(w292) -> ()
              n144 = call "controlAQuadBInResolution.vi"("Set"=FALSE, "error in"=w276, "axis in"=w268, "connection ID"=w260) -> ("error out"=w277:errorcluster, "Resolution out"=w291:i32, "axis out"=w269:u8, "connection ID"=w261:refnum<k5>)  [unwired: 3 in]
              n145 = local write "AquadB in res 2"(w291) -> ()
              n146 = call "controlAQuadBOut.vi"("Set"=FALSE, "error in"=w277, "axis in"=w269, "connection ID"=w261) -> ("error out"=w278:errorcluster, "ABout out"=w290:bool, "axis out"=w270:u8, "connection ID"=w262:refnum<k5>)  [unwired: 4 in]
              n147 = local write "AquadB out 2"(w290) -> ()
              n148 = call "controlAQuadBOutClock.vi"("Set"=FALSE, "error in"=w278, "axis in"=w270, "connection ID"=w262) -> ("error out"=w279:errorcluster, "clock out"=w289:i32, "axis out"=w271:u8, "connection ID"=w263:refnum<k5>)  [unwired: 4 in]
              n149 = local write "AqaudB clock 2"(w289) -> ()
              n150 = call "controlAQuadBOutResolution.vi"("Set"=FALSE, "error in"=w279, "axis in"=w271, "connection ID"=w263) -> ("ABoutRes out"=w288:i32)  [unwired: 4 in, 3 out]
              n151 = local write "AquadB Resolution 2"(w288) -> ()
            }
            frame #7 {
              w299 = u8 2 items=["1", "2", "3"] ("axis")
              # "get Realtime Configuration Parameters Axis 3"
              n152 = call "controlRealtimeInputMode.vi"("Set"=FALSE, "axis in"=w299, "connection ID"=w341) -> ("error out"=w316:errorcluster, "RT Mode out"=w340:i32, "axis out"=w308:u8, "connection ID"=w300:refnum<k5>)  [unwired: 5 in]
              n153 = local write "Mode Input 3"(w340) -> ()
              n154 = call "controlRealtimeInputLoopMode.vi"("Set"=FALSE, "error in"=w316, "axis in"=w308, "connection ID"=w300) -> ("error out"=w317:errorcluster, "RT Loop out"=w339:i32, "axis out"=w309:u8, "connection ID"=w301:refnum<k5>)  [unwired: 4 in]
              n155 = local write "Loop Mode 3"(w339) -> ()
              n156 = call "controlRealtimeInputStepsPerPulse.vi"("Set"=FALSE, "error in"=w317, "axis in"=w309, "connection ID"=w301) -> ("error out"=w318:errorcluster, "Steps out"=w338:i32, "axis out"=w310:u8, "connection ID"=w302:refnum<k5>)  [unwired: 4 in]
              n157 = local write "Steps per pulse 3"(w338) -> ()
              n158 = call "controlRealTimeInChangePerPulse.vi"("Set"=FALSE, "error in"=w318, "axis in"=w310, "connection ID"=w302) -> ("error out"=w319:errorcluster, "Change out"=w337:i32, "axis out"=w311:u8, "connection ID"=w303:refnum<k5>)  [unwired: 4 in]
              n159 = local write "Change per pulse 3"(w337) -> ()
              n160 = call "controlRealtimeInputMove.vi"("Set"=FALSE, "error in"=w319, "axis in"=w311, "connection ID"=w303) -> ("error out"=w320:errorcluster, "move out"=w336:bool, "axis out"=w312:u8, "connection ID"=w304:refnum<k5>)  [unwired: 4 in]
              n161 = local write "RT in move Signal 3"(w336) -> ()
              n162 = local write "RT in move 3"(w336) -> ()
              n163 = call "controlAQuadBInResolution.vi"("Set"=FALSE, "error in"=w320, "axis in"=w312, "connection ID"=w304) -> ("error out"=w321:errorcluster, "Resolution out"=w335:i32, "axis out"=w313:u8, "connection ID"=w305:refnum<k5>)  [unwired: 3 in]
              n164 = local write "AquadB in res 3"(w335) -> ()
              n165 = call "controlAQuadBOut.vi"("Set"=FALSE, "error in"=w321, "axis in"=w313, "connection ID"=w305) -> ("error out"=w322:errorcluster, "ABout out"=w334:bool, "axis out"=w314:u8, "connection ID"=w306:refnum<k5>)  [unwired: 4 in]
              n166 = local write "AquadB out 3"(w334) -> ()
              n167 = call "controlAQuadBOutClock.vi"("Set"=FALSE, "error in"=w322, "axis in"=w314, "connection ID"=w306) -> ("error out"=w323:errorcluster, "clock out"=w333:i32, "axis out"=w315:u8, "connection ID"=w307:refnum<k5>)  [unwired: 4 in]
              n168 = local write "AqaudB clock 3"(w333) -> ()
              n169 = call "controlAQuadBOutResolution.vi"("Set"=FALSE, "error in"=w323, "axis in"=w315, "connection ID"=w307) -> ("ABoutRes out"=w332:i32)  [unwired: 4 in, 3 out]
              n170 = local write "AquadB Resolution 3"(w332) -> ()
            }
          }
        }
        frame #1 {
          # "Main Loop"
          n171 = while {
            tunnel: w342 -> [w343]
            stop <- "stop" stop-if-true
            n172 = case shown="\"Navigation\", Default" "Tab Control" {
              tunnel: w343 -> [w346 w916 w1304]
              frame "Navigation", Default {
                n173 = stacked-sequence {
                  tunnel: w346 -> [w347 w536 w726]
                  frame #0 {
                    w353 = u8 0 items=["1", "2", "3"] ("axis in")
                    # "update Axis 1"
                    n174 = event shown="[17] Timeout" {
                      selector: _ -> [_ _ _ _ _ _ _ _ _ _ _ _ _ _ _ _ _ _]
                      dyn-events: _ -> [_ _ _ _ _ _ _ _ _ _ _ _ _ _ _ _ _ _]
                      timeout: 10 -> [_ _ _ _ _ _ _ _ _ _ _ _ _ _ _ _ _ _]
                      tunnel: w353 -> [w359 w370 _ w388 w397 w403 w412 w419 w424 w429 w440 w452 _ w464 w472 w483 w491 w520]
                      tunnel: [w356 w366 w376 w385 w395 w401 w410 w417 w422 w427 w438 w449 _ w461 w469 w479 w489 w502] -> w351
                      tunnel: w347 -> [w360 w371 w379 w389 w398 w404 w413 w420 w425 w430 w441 w453 _ w465 w473 w484 w493 w521]
                      event "Amplitude [V]": Value Change {
                        n175 = event-data() -> ()  [unwired: 1 in, 1 out]
                        n176 = call "ControlAmplitude.vi"("Set"=TRUE, "amplitude [V] in"="Amplitude [V]", "axis in"=w359, "connection ID"=w360) -> ("error out"=w361:errorcluster, "axis out"=w363:u8, "connection ID"=w364:refnum<k5>)  [unwired: 4 in, 1 out]
                        n177 = call "ControlAmplitude.vi"("Set"=FALSE, "error in"=w361, "axis in"=w363, "connection ID"=w364) -> ("error out"=w356:errorcluster, "amplitude [V] out"=w357:dbl)  [unwired: 4 in, 2 out]
                        n178 = local write "Amplitude [V]"(w357) -> ()
                      }
                      event "Output": Value Change {
                        n179 = event-data() -> ()  [unwired: 1 in, 1 out]
                        n180 = call "ControlOutput.vi"("Set"=TRUE, "enable output in"="Output", "axis in"=w370, "connection ID"=w371) -> ("error out"=w367:errorcluster, "axis out"=w372:u8, "connection ID"=w373:refnum<k5>)  [unwired: 4 in, 1 out]
                        n181 = call "ControlOutput.vi"("Set"=FALSE, "error in"=w367, "axis in"=w372, "connection ID"=w373) -> ("error out"=w366:errorcluster, "enable output out"=→"Output Status 1":bool)  [unwired: 4 in, 2 out]
                      }
                      event "Frequency [Hz]": Value Change {
                        n182 = event-data() -> ()  [unwired: 1 in, 1 out]
                        n183 = call "ControlFrequency.vi"("Set"=TRUE, "Frequency [Hz] in"="Frequency [Hz]", "connection ID"=w379) -> ("error out"=w380:errorcluster, "axis out"=w381:u8, "connection ID"=w384:refnum<k5>)  [unwired: 5 in, 1 out]
                        n184 = call "ControlFrequency.vi"("Set"=FALSE, "error in"=w380, "axis in"=w381, "connection ID"=w384) -> ("error out"=w376:errorcluster, "Frequency [Hz] out"=w377:dbl)  [unwired: 4 in, 2 out]
                        n185 = local write "Frequency [Hz]"(w377) -> ()
                      }
                      event "Move": Value Change {
                        n186 = event-data() -> ()  [unwired: 1 in, 1 out]
                        n187 = call "ControlMove.vi"("Set"=TRUE, "control move in"="Move", "axis in"=w388, "connection ID"=w389) -> ("error out"=w390:errorcluster, "axis out"=w391:u8, "connection ID"=w394:refnum<k5>)  [unwired: 4 in, 1 out]
                        n188 = call "ControlMove.vi"("Set"=FALSE, "error in"=w390, "axis in"=w391, "connection ID"=w394) -> ("error out"=w385:errorcluster, "controll move out"=→"move out":bool)  [unwired: 4 in, 2 out]
                      }
                      event "EoT 1": Value Change {
                        n189 = event-data() -> ()  [unwired: 1 in, 1 out]
                        n190 = call "controlEotOutputDeactive.vi"("Set"=TRUE, "enable EOT in"="EoT 1", "axis in"=w397, "connection ID"=w398) -> ("error out"=w395:errorcluster)  [unwired: 4 in, 3 out]
                      }
                      event "Target Position 1": Value Change {
                        n191 = event-data() -> ()  [unwired: 1 in, 1 out]
                        n192 = call "ControlTargetPosition.vi"("Set"=TRUE, "Target Position in"="Target Position 1", "axis in"=w403, "connection ID"=w404) -> ("error out"=w406:errorcluster, "axis out"=w407:u8, "connection ID"=w408:refnum<k5>)  [unwired: 4 in, 1 out]
                        n193 = call "ControlTargetPosition.vi"("Set"=FALSE, "error in"=w406, "axis in"=w407, "connection ID"=w408) -> ("error out"=w401:errorcluster, "axis out"=w402:u8)  [unwired: 4 in, 2 out]
                        n194 = local write "Target Position 1"(w402) -> ()
                      }
                      event "Axis 1": Value Change {
                        n195 = event-data() -> ()  [unwired: 1 in, 1 out]
                        n196 = case shown="True" "Axis 1" {
                          tunnel: [_ w416] -> w410
                          tunnel: w413 -> [_ w415]
                          tunnel: w412 -> [_ w414]
                          frame False {
                          }
                          frame True {
                            n197 = call "setReset.vi"("axis in"=w414, "connection ID"=w415) -> ("error out"=w416:errorcluster)  [unwired: 7 in, 2 out]
                          }
                        }
                      }
                      event "Single Step Left": Value Change {
                        n198 = event-data() -> ()  [unwired: 1 in, 1 out]
                        n199 = call "setNSteps.vi"("FWD"=TRUE, "setnSteps in"="Number of steps 1", "axis in"=w419, "connection ID"=w420) -> ("error out"=w417:errorcluster)  [unwired: 4 in, 3 out]
                      }
                      event "Single Step Right": Value Change {
                        n200 = event-data() -> ()  [unwired: 1 in, 1 out]
                        n201 = local read "Number of steps 1"() -> (w423:i32)
                        n202 = call "setNSteps.vi"("FWD"=FALSE, "setnSteps in"=w423, "axis in"=w424, "connection ID"=w425) -> ("error out"=w422:errorcluster)  [unwired: 4 in, 3 out]
                      }
                      event "Endless Left": Value Change {
                        n203 = event-data() -> ()  [unwired: 1 in, 1 out]
                        n204 = call "ControlContinousFwd.vi"("Set"=TRUE, "enable in"=FALSE ("continous FWD in"), "axis in"=w429, "connection ID"=w430) -> ("error out"=w431:errorcluster, "axis out"=w435:u8, "connection ID"=w436:refnum<k5>)  [unwired: 4 in, 1 out]
                        n205 = call "ControlContinousBkwd.vi"("Set"=TRUE, "error in"=w431, "enable in"="Endless Left", "axis in"=w435, "connection ID"=w436) -> ("error out"=w427:errorcluster)  [unwired: 3 in, 3 out]
                        n206 = local write "Continuous Forward"(FALSE) -> ()
                      }
                      event "Continuous Forward": Value Change {
                        n207 = event-data() -> ()  [unwired: 1 in, 1 out]
                        n208 = call "ControlContinousBkwd.vi"("Set"=TRUE, "enable in"=FALSE ("continous BWD in"), "axis in"=w440, "connection ID"=w441) -> ("error out"=w442:errorcluster, "axis out"=w446:u8, "connection ID"=w447:refnum<k5>)  [unwired: 4 in, 1 out]
                        n209 = call "ControlContinousFwd.vi"("Set"=TRUE, "error in"=w442, "enable in"="Continuous Forward", "axis in"=w446, "connection ID"=w447) -> ("error out"=w438:errorcluster)  [unwired: 3 in, 3 out]
                        n210 = local write "Endless Left"(FALSE) -> ()
                      }
                      event "Fixed DC 1": Value Change {
                        n211 = event-data() -> ()  [unwired: 1 in, 1 out]
                        n212 = call "ControlFixOutputVoltage.vi"("Set"=TRUE, "Fixed Output Voltage in"="Fixed DC 1", "axis in"=w452, "connection ID"=w453) -> ("error out"=w454:errorcluster, "axis out"=w455:u8, "connection ID"=w456:refnum<k5>)  [unwired: 4 in, 1 out]
                        n213 = call "ControlFixOutputVoltage.vi"("Set"=FALSE, "error in"=w454, "axis in"=w455, "connection ID"=w456) -> ("error out"=w449:errorcluster, "Fixed Output Voltage out"=w450:dbl)  [unwired: 4 in, 2 out]
                        n214 = local write "Fixed DC 1"(w450) -> ()
                      }
                      event "Reset Error": Value Change {
                        n215 = event-data() -> ()  [unwired: 1 in, 1 out]
                        n216 = local write "Error Message"("" ("Error Message")) -> ()
                        n217 = local write "Error"(FALSE ("Error")) -> ()
                      }
                      event "Positioner": Value Change {
                        n218 = event-data() -> ()  [unwired: 1 in, 1 out]
                        n219 = property on="Positioner" class="Ring (strict)"() -> ("RingText.Text"=w463:string)  [unwired: 2 in, 2 out]
                        n220 = call "controlActorSelection.vi"("Positioner in"=w463, "axis in"=w464, "connection ID"=w465) -> ("error out"=w466:errorcluster, "axis out"=w467:u8, "connection ID"=w468:refnum<k5>)  [unwired: 6 in]
                        n221 = call "getActorType.vi"("error in"=w466, "axis in"=w467, "connection ID"=w468) -> ("error out"=w461:errorcluster, "Actor Type"=w462:dbl)  [unwired: 5 in, 2 out]
                        n222 = local write "actor type"(w462) -> ()
                      }
                      event "Target Range 1": Value Change {
                        n223 = event-data() -> ()  [unwired: 1 in, 1 out]
                        n224 = call "ControlTargetRange.vi"("Set"=TRUE, "Target Range in"="Target Range 1", "axis in"=w472, "connection ID"=w473) -> ("error out"=w475:errorcluster, "axis out"=w476:u8, "connection ID"=w477:refnum<k5>)  [unwired: 4 in, 1 out]
                        n225 = call "ControlTargetRange.vi"("Set"=FALSE, "error in"=w475, "axis in"=w476, "connection ID"=w477) -> ("error out"=w469:errorcluster, "Target Range out"=w470:dbl)  [unwired: 4 in, 2 out]
                        n226 = local write "Target Range 1"(w470) -> ()
                      }
                      event "auto Reset 1": Value Change {
                        n227 = event-data() -> ()  [unwired: 1 in, 1 out]
                        n228 = call "controlAutoReset.vi"("Set"=TRUE, "auto reset in"="auto Reset 1", "axis in"=w483, "connection ID"=w484) -> ("error out"=w480:errorcluster, "axis out"=w487:u8, "connection ID"=w486:refnum<k5>)  [unwired: 4 in, 1 out]
                        n229 = call "controlAutoReset.vi"("Set"=FALSE, "error in"=w480, "axis in"=w487, "connection ID"=w486) -> ("error out"=w479:errorcluster, "auto reset out"=w481:bool)  [unwired: 4 in, 2 out]
                        n230 = local write "auto Reset 1"(w481) -> ()
                      }
                      event "Reference Auto Update 1": Value Change {
                        n231 = event-data() -> ()  [unwired: 1 in, 1 out]
                        n232 = call "controlReferenceAutoUpdate.vi"("Set"=TRUE, "ref auto up in"="Reference Auto Update 1", "axis in"=w491, "connection ID"=w493) -> ("error out"=w498:errorcluster, "axis out"=w497:u8, "connection ID"=w496:refnum<k5>)  [unwired: 4 in, 1 out]
                        n233 = call "controlReferenceAutoUpdate.vi"("Set"=FALSE, "error in"=w498, "axis in"=w497, "connection ID"=w496) -> ("error out"=w489:errorcluster, "ref auto up out"=w490:bool)  [unwired: 4 in, 2 out]
                        n234 = local write "Reference Auto Update 1"(w490) -> ()
                      }
                      event Timeout {
                        n235 = event-data() -> ()  [unwired: 1 in, 1 out]
                        n236 = call "getPosition.vi"("axis in"=w520, "connection ID"=w521) -> ("error out"=w512:errorcluster, "position out"=→"Position":dbl, "axis out"=w534:u8, "connection ID"=w535:refnum<k5>)  [unwired: 6 in]
                        n237 = call "getReferencePosition.vi"("error in"=w512, "axis in"=w534, "connection ID"=w535) -> ("error out"=w511:errorcluster, "Reference position out"=→"Reference":dbl, "axis out"=w532:u8, "connection ID"=w533:refnum<k5>)  [unwired: 5 in]
                        n238 = call "getStatusConnected.vi"("error in"=w511, "axis in"=w532, "connection ID"=w533) -> ("error out"=w510:errorcluster, "Status Connected out"=→"Connected":bool, "axis out"=w530:u8, "connection ID"=w531:refnum<k5>)  [unwired: 5 in]
                        n239 = call "getStatusMoving.vi"("error in"=w510, "axis in"=w530, "connection ID"=w531) -> ("error out"=w509:errorcluster, "status moving out"=→"MoveSignal":bool, "axis out"=w528:u8, "connection ID"=w529:refnum<k5>)  [unwired: 5 in]
                        n240 = call "getStatusReference.vi"("error in"=w509, "axis in"=w528, "connection ID"=w529) -> ("error out"=w508:errorcluster, "status reference out"=→"ReferenceSignal":bool, "axis out"=w526:u8, "connection ID"=w527:refnum<k5>)  [unwired: 5 in]
                        n241 = call "getStatusEotBkwd.vi"("error in"=w508, "axis in"=w526, "connection ID"=w527) -> ("error out"=w507:errorcluster, "Get Stus EOT BKWD out"=→"EotLeftDetected1":bool, "axis out"=w524:u8, "connection ID"=w525:refnum<k5>)  [unwired: 5 in]
                        n242 = call "getStatusEotFwd.vi"("error in"=w507, "axis in"=w524, "connection ID"=w525) -> ("error out"=w506:errorcluster, "Status EOT FWD out"=→"EotrightDetected1":bool, "axis out"=w522:u8, "connection ID"=w523:refnum<k5>)  [unwired: 5 in]
                        n243 = call "getStatusTargetRange.vi"("error in"=w506, "axis in"=w522, "connection ID"=w523) -> ("error out"=w503:errorcluster, "Status Target Range out"=→"in target range1":bool, "axis out"=w504:u8, "connection ID"=w505:refnum<k5>)  [unwired: 5 in]
                        n244 = call "ControlMove.vi"("Set"=FALSE, "error in"=w503, "axis in"=w504, "connection ID"=w505) -> ("error out"=w502:errorcluster, "controll move out"=w500:bool)  [unwired: 4 in, 2 out]
                        n245 = local write "Move"(w500) -> ()
                        n246 = local write "move out"(w500) -> ()
                      }
                    }
                    n247 = Unbundle(w351) -> ("code"=w349:i32, "source"=w350:string)  [unwired: 1 out]
                    n248 = Not Equal To 0?(x=w349) -> (x != 0?=w348:bool)
                    n249 = case shown="True" w348 {
                      selector: w348 -> [_ w354]
                      tunnel: w350 -> [_ w355]
                      frame False {
                      }
                      frame True {
                        "Error Message" <- w355
                        "Error" <- w354
                      }
                    }
                  }
                  frame #1 {
                    w542 = u8 1 items=["1", "2", "3"] ("axis in")
                    # "update Axis 2"
                    n250 = event shown="[11] \"Fixed DC 2\": Value Change" {
                      selector: _ -> [_ _ _ _ _ _ _ _ _ _ _ _ _ _ _ _ _ _]
                      dyn-events: _ -> [_ _ _ _ _ _ _ _ _ _ _ _ _ _ _ _ _ _]
                      timeout: 10 -> [_ _ _ _ _ _ _ _ _ _ _ _ _ _ _ _ _ _]
                      tunnel: w542 -> [w551 w562 w570 w580 w588 w598 w601 w610 w615 w624 w635 w644 _ w656 w665 w677 w687 w706]
                      tunnel: [w545 w557 w565 w575 w585 w593 w600 w608 w612 w617 w629 w641 _ w651 w661 w669 w679 w694] -> w539
                      tunnel: w536 -> [w554 w564 w574 w584 w589 w599 w602 w611 w616 w626 w637 w648 _ w658 w668 w678 w688 w725]
                      event "amplitude [V] 2": Value Change {
                        n251 = event-data() -> ()  [unwired: 1 in, 1 out]
                        n252 = call "ControlAmplitude.vi"("Set"=TRUE, "amplitude [V] in"="amplitude [V] 2", "axis in"=w551, "connection ID"=w554) -> ("error out"=w546:errorcluster, "axis out"=w550:u8, "connection ID"=w552:refnum<k5>)  [unwired: 4 in, 1 out]
                        n253 = call "ControlAmplitude.vi"("Set"=FALSE, "error in"=w546, "axis in"=w550, "connection ID"=w552) -> ("error out"=w545:errorcluster, "amplitude [V] out"=w547:dbl)  [unwired: 4 in, 2 out]
                        n254 = local write "amplitude [V] 2"(w547) -> ()
                      }
                      event "Output 2": Value Change {
                        n255 = event-data() -> ()  [unwired: 1 in, 1 out]
                        n256 = call "ControlOutput.vi"("Set"=TRUE, "enable output in"="Output 2", "axis in"=w562, "connection ID"=w564) -> ("error out"=w555:errorcluster, "axis out"=w558:u8, "connection ID"=w559:refnum<k5>)  [unwired: 4 in, 1 out]
                        n257 = call "ControlOutput.vi"("Set"=FALSE, "error in"=w555, "axis in"=w558, "connection ID"=w559) -> ("error out"=w557:errorcluster, "enable output out"=→"Output Status 2":bool)  [unwired: 4 in, 2 out]
                      }
                      event "frequency [Hz] 2": Value Change {
                        n258 = event-data() -> ()  [unwired: 1 in, 1 out]
                        n259 = call "ControlFrequency.vi"("Set"=TRUE, "Frequency [Hz] in"="frequency [Hz] 2", "axis in"=w570, "connection ID"=w574) -> ("error out"=w566:errorcluster, "axis out"=w569:u8, "connection ID"=w573:refnum<k5>)  [unwired: 4 in, 1 out]
                        n260 = call "ControlFrequency.vi"("Set"=FALSE, "error in"=w566, "axis in"=w569, "connection ID"=w573) -> ("error out"=w565:errorcluster, "Frequency [Hz] out"=w568:dbl)  [unwired: 4 in, 2 out]
                        n261 = local write "frequency [Hz] 2"(w568) -> ()
                      }
                      event "Move 2": Value Change {
                        n262 = event-data() -> ()  [unwired: 1 in, 1 out]
                        n263 = call "ControlMove.vi"("Set"=TRUE, "control move in"="Move 2", "axis in"=w580, "connection ID"=w584) -> ("error out"=w576:errorcluster, "axis out"=w579:u8, "connection ID"=w583:refnum<k5>)  [unwired: 4 in, 1 out]
                        n264 = call "ControlMove.vi"("Set"=FALSE, "error in"=w576, "axis in"=w579, "connection ID"=w583) -> ("error out"=w575:errorcluster, "controll move out"=→"move out 2":bool)  [unwired: 4 in, 2 out]
                      }
                      event "EoT 2": Value Change {
                        n265 = event-data() -> ()  [unwired: 1 in, 1 out]
                        n266 = call "controlEotOutputDeactive.vi"("Set"=TRUE, "enable EOT in"="EoT 2", "axis in"=w588, "connection ID"=w589) -> ("error out"=w585:errorcluster)  [unwired: 4 in, 3 out]
                      }
                      event "Target position 2": Value Change {
                        n267 = event-data() -> ()  [unwired: 1 in, 1 out]
                        n268 = call "ControlTargetPosition.vi"("Set"=TRUE, "Target Position in"="Target position 2", "axis in"=w598, "connection ID"=w599) -> ("error out"=w594:errorcluster, "axis out"=w595:u8, "connection ID"=w596:refnum<k5>)  [unwired: 4 in, 1 out]
                        n269 = call "ControlTargetPosition.vi"("Set"=FALSE, "error in"=w594, "axis in"=w595, "connection ID"=w596) -> ("error out"=w593:errorcluster, "Target Position out"=w591:dbl)  [unwired: 4 in, 2 out]
                        n270 = local write "Target position 2"(w591) -> ()
                      }
                      event "Axis 2": Value Change {
                        n271 = event-data() -> ()  [unwired: 1 in, 1 out]
                        n272 = case shown="True" "Axis 2" {
                          tunnel: w602 -> [_ w606]
                          tunnel: w601 -> [_ w605]
                          tunnel: [_ w604] -> w600
                          frame False {
                          }
                          frame True {
                            n273 = call "setReset.vi"("axis in"=w605, "connection ID"=w606) -> ("error out"=w604:errorcluster)  [unwired: 7 in, 2 out]
                          }
                        }
                      }
                      event "Single Step Left 2": Value Change {
                        n274 = event-data() -> ()  [unwired: 1 in, 1 out]
                        n275 = call "setNSteps.vi"("FWD"=TRUE, "setnSteps in"="Number of steps 2", "axis in"=w610, "connection ID"=w611) -> ("error out"=w608:errorcluster)  [unwired: 4 in, 3 out]
                      }
                      event "Single Step Right 2": Value Change {
                        n276 = event-data() -> ()  [unwired: 1 in, 1 out]
                        n277 = local read "Number of steps 2"() -> (w614:i32)
                        n278 = call "setNSteps.vi"("FWD"=FALSE, "setnSteps in"=w614, "axis in"=w615, "connection ID"=w616) -> ("error out"=w612:errorcluster)  [unwired: 4 in, 3 out]
                      }
                      event "Endless Left 2": Value Change {
                        n279 = event-data() -> ()  [unwired: 1 in, 1 out]
                        n280 = call "ControlContinousFwd.vi"("Set"=TRUE, "enable in"=FALSE ("continous FWD in"), "axis in"=w624, "connection ID"=w626) -> ("error out"=w618:errorcluster, "axis out"=w623:u8, "connection ID"=w625:refnum<k5>)  [unwired: 4 in, 1 out]
                        n281 = call "ControlContinousBkwd.vi"("Set"=TRUE, "error in"=w618, "enable in"="Endless Left 2", "axis in"=w623, "connection ID"=w625) -> ("error out"=w617:errorcluster)  [unwired: 3 in, 3 out]
                        n282 = local write "Continuous Forward"(FALSE) -> ()
                      }
                      event "Continuous Forward": Value Change {
                        n283 = event-data() -> ()  [unwired: 1 in, 1 out]
                        n284 = call "ControlContinousBkwd.vi"("Set"=TRUE, "enable in"=FALSE ("continous BWD in"), "axis in"=w635, "connection ID"=w637) -> ("error out"=w630:errorcluster, "axis out"=w634:u8, "connection ID"=w636:refnum<k5>)  [unwired: 4 in, 1 out]
                        n285 = call "ControlContinousFwd.vi"("Set"=TRUE, "error in"=w630, "enable in"="Continuous Forward", "axis in"=w634, "connection ID"=w636) -> ("error out"=w629:errorcluster)  [unwired: 3 in, 3 out]
                        n286 = local write "Endless Left 2"(FALSE ("Endless Left 2")) -> ()
                      }
                      event "Fixed DC 2": Value Change {
                        n287 = event-data() -> ()  [unwired: 1 in, 1 out]
                        n288 = call "ControlFixOutputVoltage.vi"("Set"=TRUE, "Fixed Output Voltage in"="Fixed DC 2", "axis in"=w644, "connection ID"=w648) -> ("error out"=w642:errorcluster, "axis out"=w643:u8, "connection ID"=w645:refnum<k5>)  [unwired: 4 in, 1 out]
                        n289 = call "ControlFixOutputVoltage.vi"("Set"=FALSE, "error in"=w642, "axis in"=w643, "connection ID"=w645) -> ("error out"=w641:errorcluster, "Fixed Output Voltage out"=w639:dbl)  [unwired: 4 in, 2 out]
                        n290 = local write "Fixed DC 2"(w639) -> ()
                      }
                      event "Reset Error 2": Value Change {
                        n291 = event-data() -> ()  [unwired: 1 in, 1 out]
                        n292 = local write "Error Message 2"("" ("Error Message 2")) -> ()
                        n293 = local write "Error 2"(FALSE ("Error 2")) -> ()
                      }
                      event "Positioner 2": Value Change {
                        n294 = event-data() -> ()  [unwired: 1 in, 1 out]
                        n295 = property on="Positioner 2" class="Ring (strict)"() -> ("RingText.Text"=w657:string)  [unwired: 2 in, 2 out]
                        n296 = call "controlActorSelection.vi"("Positioner in"=w657, "axis in"=w656, "connection ID"=w658) -> ("error out"=w652:errorcluster, "axis out"=w654:u8, "connection ID"=w655:refnum<k5>)  [unwired: 6 in]
                        n297 = call "getActorType.vi"("error in"=w652, "axis in"=w654, "connection ID"=w655) -> ("error out"=w651:errorcluster, "Actor Type"=w653:dbl)  [unwired: 5 in, 2 out]
                        n298 = local write "actor type 2"(w653) -> ()
                      }
                      event "Target Range 2": Value Change {
                        n299 = event-data() -> ()  [unwired: 1 in, 1 out]
                        n300 = call "ControlTargetRange.vi"("Set"=TRUE, "Target Range in"="Target Range 2", "axis in"=w665, "connection ID"=w668) -> ("error out"=w662:errorcluster, "axis out"=w663:u8, "connection ID"=w664:refnum<k5>)  [unwired: 4 in, 1 out]
                        n301 = call "ControlTargetRange.vi"("Set"=FALSE, "error in"=w662, "axis in"=w663, "connection ID"=w664) -> ("error out"=w661:errorcluster, "Target Range out"=w660:dbl)  [unwired: 4 in, 2 out]
                        n302 = local write "Target Range 2"(w660) -> ()
                      }
                      event "auto Reset 2": Value Change {
                        n303 = event-data() -> ()  [unwired: 1 in, 1 out]
                        n304 = call "controlAutoReset.vi"("Set"=TRUE, "auto reset in"="auto Reset 2", "axis in"=w677, "connection ID"=w678) -> ("error out"=w670:errorcluster, "axis out"=w674:u8, "connection ID"=w675:refnum<k5>)  [unwired: 4 in, 1 out]
                        n305 = call "controlAutoReset.vi"("Set"=FALSE, "error in"=w670, "axis in"=w674, "connection ID"=w675) -> ("error out"=w669:errorcluster, "auto reset out"=w671:bool)  [unwired: 4 in, 2 out]
                        n306 = local write "auto Reset 2"(w671) -> ()
                      }
                      event "Reference Auto Update 2": Value Change {
                        n307 = event-data() -> ()  [unwired: 1 in, 1 out]
                        n308 = call "controlReferenceAutoUpdate.vi"("Set"=TRUE, "ref auto up in"="Reference Auto Update 2", "axis in"=w687, "connection ID"=w688) -> ("error out"=w682:errorcluster, "axis out"=w683:u8, "connection ID"=w684:refnum<k5>)  [unwired: 4 in, 1 out]
                        n309 = call "controlReferenceAutoUpdate.vi"("Set"=FALSE, "error in"=w682, "axis in"=w683, "connection ID"=w684) -> ("error out"=w679:errorcluster, "ref auto up out"=w680:bool)  [unwired: 4 in, 2 out]
                        n310 = local write "Reference Auto Update 2"(w680) -> ()
                      }
                      event Timeout {
                        n311 = event-data() -> ()  [unwired: 1 in, 1 out]
                        n312 = call "getPosition.vi"("axis in"=w706, "connection ID"=w725) -> ("error out"=w702:errorcluster, "position out"=→"Position 2":dbl, "axis out"=w722:u8, "connection ID"=w723:refnum<k5>)  [unwired: 6 in]
                        n313 = call "getReferencePosition.vi"("error in"=w702, "axis in"=w722, "connection ID"=w723) -> ("error out"=w701:errorcluster, "Reference position out"=→"Reference 2":dbl, "axis out"=w719:u8, "connection ID"=w720:refnum<k5>)  [unwired: 5 in]
                        n314 = call "getStatusConnected.vi"("error in"=w701, "axis in"=w719, "connection ID"=w720) -> ("error out"=w700:errorcluster, "Status Connected out"=→"Connected 2":bool, "axis out"=w716:u8, "connection ID"=w717:refnum<k5>)  [unwired: 5 in]
                        n315 = call "getStatusMoving.vi"("error in"=w700, "axis in"=w716, "connection ID"=w717) -> ("error out"=w699:errorcluster, "status moving out"=→"MoveSignal 2":bool, "axis out"=w713:u8, "connection ID"=w714:refnum<k5>)  [unwired: 5 in]
                        n316 = call "getStatusReference.vi"("error in"=w699, "axis in"=w713, "connection ID"=w714) -> ("error out"=w698:errorcluster, "status reference out"=→"ReferenceSignal 2":bool, "axis out"=w710:u8, "connection ID"=w711:refnum<k5>)  [unwired: 5 in]
                        n317 = call "getStatusEotBkwd.vi"("error in"=w698, "axis in"=w710, "connection ID"=w711) -> ("error out"=w697:errorcluster, "Get Stus EOT BKWD out"=→"EotLeftDetected2":bool, "axis out"=w708:u8, "connection ID"=w709:refnum<k5>)  [unwired: 5 in]
                        n318 = call "getStatusEotFwd.vi"("error in"=w697, "axis in"=w708, "connection ID"=w709) -> ("error out"=w696:errorcluster, "Status EOT FWD out"=→"EotrightDetected2":bool, "axis out"=w703:u8, "connection ID"=w704:refnum<k5>)  [unwired: 5 in]
                        n319 = call "getStatusTargetRange.vi"("error in"=w696, "axis in"=w703, "connection ID"=w704) -> ("error out"=w695:errorcluster, "Status Target Range out"=→"in target range2":bool, "axis out"=w691:u8, "connection ID"=w692:refnum<k5>)  [unwired: 5 in]
                        n320 = call "ControlMove.vi"("Set"=FALSE, "error in"=w695, "axis in"=w691, "connection ID"=w692) -> ("error out"=w694:errorcluster, "controll move out"=w690:bool)  [unwired: 4 in, 2 out]
                        n321 = local write "move out 2"(w690) -> ()
                        n322 = local write "Move 2"(w690) -> ()
                      }
                    }
                    n323 = Unbundle(w539) -> ("code"=w538:i32, "source"=w540:string)  [unwired: 1 out]
                    n324 = Not Equal To 0?(x=w538) -> (x != 0?=w537:bool)
                    n325 = case shown="False" w537 {
                      selector: w537 -> [_ w543]
                      tunnel: w540 -> [_ w544]
                      frame False {
                      }
                      frame True {
                        "Error Message 2" <- w544
                        "Error 2" <- w543
                      }
                    }
                  }
                  frame #2 {
                    w732 = u8 2 items=["1", "2", "3"] ("axis in")
                    # "update Axis 3"
                    n326 = event shown="[13] \"Positioner 3\": Value Change" {
                      selector: _ -> [_ _ _ _ _ _ _ _ _ _ _ _ _ _ _ _ _ _]
                      dyn-events: _ -> [_ _ _ _ _ _ _ _ _ _ _ _ _ _ _ _ _ _]
                      timeout: 10 -> [_ _ _ _ _ _ _ _ _ _ _ _ _ _ _ _ _ _]
                      tunnel: w732 -> [w738 w749 w758 w768 w777 w783 w792 w799 w804 w809 w820 w831 _ w844 w852 w863 w871 w899]
                      tunnel: [w735 w745 w755 w765 w775 w781 w790 w797 w802 w807 w818 w829 _ w842 w849 w859 w869 w881] -> w729
                      tunnel: w726 -> [w739 w750 w759 w769 w778 w784 w793 w800 w805 w810 w821 w833 _ w845 w853 w864 w873 w900]
                      event "amplitude [V] 3": Value Change {
                        n327 = event-data() -> ()  [unwired: 1 in, 1 out]
                        n328 = call "ControlAmplitude.vi"("Set"=TRUE, "amplitude [V] in"="amplitude [V] 3", "axis in"=w738, "connection ID"=w739) -> ("error out"=w740:errorcluster, "axis out"=w742:u8, "connection ID"=w743:refnum<k5>)  [unwired: 4 in, 1 out]
                        n329 = call "ControlAmplitude.vi"("Set"=FALSE, "error in"=w740, "axis in"=w742, "connection ID"=w743) -> ("error out"=w735:errorcluster, "amplitude [V] out"=w736:dbl)  [unwired: 4 in, 2 out]
                        n330 = local write "amplitude [V] 3"(w736) -> ()
                      }
                      event "Output 3": Value Change {
                        n331 = event-data() -> ()  [unwired: 1 in, 1 out]
                        n332 = call "ControlOutput.vi"("Set"=TRUE, "enable output in"="Output 3", "axis in"=w749, "connection ID"=w750) -> ("error out"=w746:errorcluster, "axis out"=w751:u8, "connection ID"=w752:refnum<k5>)  [unwired: 4 in, 1 out]
                        n333 = call "ControlOutput.vi"("Set"=FALSE, "error in"=w746, "axis in"=w751, "connection ID"=w752) -> ("error out"=w745:errorcluster, "enable output out"=→"Output Satus 3":bool)  [unwired: 4 in, 2 out]
                      }
                      event "frequency [Hz] 3": Value Change {
                        n334 = event-data() -> ()  [unwired: 1 in, 1 out]
                        n335 = call "ControlFrequency.vi"("Set"=TRUE, "Frequency [Hz] in"="frequency [Hz] 3", "axis in"=w758, "connection ID"=w759) -> ("error out"=w760:errorcluster, "axis out"=w761:u8, "connection ID"=w764:refnum<k5>)  [unwired: 4 in, 1 out]
                        n336 = call "ControlFrequency.vi"("Set"=FALSE, "error in"=w760, "axis in"=w761, "connection ID"=w764) -> ("error out"=w755:errorcluster, "Frequency [Hz] out"=w756:dbl)  [unwired: 4 in, 2 out]
                        n337 = local write "frequency [Hz] 3"(w756) -> ()
                      }
                      event "Move 3": Value Change {
                        n338 = event-data() -> ()  [unwired: 1 in, 1 out]
                        n339 = call "ControlMove.vi"("Set"=TRUE, "control move in"="Move 3", "axis in"=w768, "connection ID"=w769) -> ("error out"=w770:errorcluster, "axis out"=w771:u8, "connection ID"=w774:refnum<k5>)  [unwired: 4 in, 1 out]
                        n340 = call "ControlMove.vi"("Set"=FALSE, "error in"=w770, "axis in"=w771, "connection ID"=w774) -> ("error out"=w765:errorcluster, "controll move out"=→"move out 3":bool)  [unwired: 4 in, 2 out]
                      }
                      event "EoT 3": Value Change {
                        n341 = event-data() -> ()  [unwired: 1 in, 1 out]
                        n342 = call "controlEotOutputDeactive.vi"("Set"=TRUE, "enable EOT in"="EoT 3", "axis in"=w777, "connection ID"=w778) -> ("error out"=w775:errorcluster)  [unwired: 4 in, 3 out]
                      }
                      event "Target Position 3": Value Change {
                        n343 = event-data() -> ()  [unwired: 1 in, 1 out]
                        n344 = call "ControlTargetPosition.vi"("Set"=TRUE, "Target Position in"="Target Position 3", "axis in"=w783, "connection ID"=w784) -> ("error out"=w786:errorcluster, "axis out"=w787:u8, "connection ID"=w788:refnum<k5>)  [unwired: 4 in, 1 out]
                        n345 = call "ControlTargetPosition.vi"("Set"=FALSE, "error in"=w786, "axis in"=w787, "connection ID"=w788) -> ("error out"=w781:errorcluster, "axis out"=w782:u8)  [unwired: 4 in, 2 out]
                        n346 = local write "Target Position 3"(w782) -> ()
                      }
                      event "Axis 3": Value Change {
                        n347 = event-data() -> ()  [unwired: 1 in, 1 out]
                        n348 = case shown="True" "Axis 3" {
                          tunnel: [_ w796] -> w790
                          tunnel: w793 -> [_ w795]
                          tunnel: w792 -> [_ w794]
                          frame False {
                          }
                          frame True {
                            n349 = call "setReset.vi"("axis in"=w794, "connection ID"=w795) -> ("error out"=w796:errorcluster)  [unwired: 7 in, 2 out]
                          }
                        }
                      }
                      event "Single Step Left 3": Value Change {
                        n350 = event-data() -> ()  [unwired: 1 in, 1 out]
                        n351 = call "setNSteps.vi"("FWD"=TRUE, "setnSteps in"="Number of steps 3", "axis in"=w799, "connection ID"=w800) -> ("error out"=w797:errorcluster)  [unwired: 4 in, 3 out]
                      }
                      event "Single Step Right 3": Value Change {
                        n352 = event-data() -> ()  [unwired: 1 in, 1 out]
                        n353 = local read "Number of steps 3"() -> (w803:i32)
                        n354 = call "setNSteps.vi"("FWD"=FALSE, "setnSteps in"=w803, "axis in"=w804, "connection ID"=w805) -> ("error out"=w802:errorcluster)  [unwired: 4 in, 3 out]
                      }
                      event "Endless Left 3": Value Change {
                        n355 = event-data() -> ()  [unwired: 1 in, 1 out]
                        n356 = call "ControlContinousFwd.vi"("Set"=TRUE, "enable in"=FALSE ("continous FWD in"), "axis in"=w809, "connection ID"=w810) -> ("error out"=w811:errorcluster, "axis out"=w815:u8, "connection ID"=w816:refnum<k5>)  [unwired: 4 in, 1 out]
                        n357 = call "ControlContinousBkwd.vi"("Set"=TRUE, "error in"=w811, "enable in"="Endless Left 3", "axis in"=w815, "connection ID"=w816) -> ("error out"=w807:errorcluster)  [unwired: 3 in, 3 out]
                        n358 = local write "Continuous Forward"(FALSE ("Endless Right 3")) -> ()
                      }
                      event "Continuous Forward": Value Change {
                        n359 = event-data() -> ()  [unwired: 1 in, 1 out]
                        n360 = call "ControlContinousBkwd.vi"("Set"=TRUE, "enable in"=FALSE ("continous BWD in"), "axis in"=w820, "connection ID"=w821) -> ("error out"=w822:errorcluster, "axis out"=w826:u8, "connection ID"=w827:refnum<k5>)  [unwired: 4 in, 1 out]
                        n361 = call "ControlContinousFwd.vi"("Set"=TRUE, "error in"=w822, "enable in"="Continuous Forward", "axis in"=w826, "connection ID"=w827) -> ("error out"=w818:errorcluster)  [unwired: 3 in, 3 out]
                        n362 = local write "Endless Left 3"(FALSE ("Endless Left 3")) -> ()
                      }
                      event "Fixed DC 3": Value Change {
                        n363 = event-data() -> ()  [unwired: 1 in, 1 out]
                        n364 = call "ControlFixOutputVoltage.vi"("Set"=TRUE, "Fixed Output Voltage in"="Fixed DC 3", "axis in"=w831, "connection ID"=w833) -> ("error out"=w834:errorcluster, "axis out"=w835:u8, "connection ID"=w836:refnum<k5>)  [unwired: 4 in, 1 out]
                        n365 = call "ControlFixOutputVoltage.vi"("Set"=FALSE, "error in"=w834, "axis in"=w835, "connection ID"=w836) -> ("error out"=w829:errorcluster, "Fixed Output Voltage out"=w830:dbl)  [unwired: 4 in, 2 out]
                        n366 = local write "Fixed DC 3"(w830) -> ()
                      }
                      event "Reset Error 3": Value Change {
                        n367 = event-data() -> ()  [unwired: 1 in, 1 out]
                        n368 = local write "Error Message 3"("" ("Error Message 3")) -> ()
                        n369 = local write "Error 3"(FALSE ("Error 3")) -> ()
                      }
                      event "Positioner 3": Value Change {
                        n370 = event-data() -> ()  [unwired: 1 in, 1 out]
                        n371 = property on="Positioner 3" class="Ring (strict)"() -> ("RingText.Text"=w843:string)  [unwired: 2 in, 2 out]
                        n372 = call "controlActorSelection.vi"("Positioner in"=w843, "axis in"=w844, "connection ID"=w845) -> ("error out"=w846:errorcluster, "axis out"=w847:u8, "connection ID"=w848:refnum<k5>)  [unwired: 6 in]
                        n373 = call "getActorType.vi"("error in"=w846, "axis in"=w847, "connection ID"=w848) -> ("error out"=w842:errorcluster, "Actor Type"=w841:dbl)  [unwired: 5 in, 2 out]
                        n374 = local write "actor type 3"(w841) -> ()
                      }
                      event "Target Range 3": Value Change {
                        n375 = event-data() -> ()  [unwired: 1 in, 1 out]
                        n376 = call "ControlTargetRange.vi"("Set"=TRUE, "Target Range in"="Target Range 3", "axis in"=w852, "connection ID"=w853) -> ("error out"=w855:errorcluster, "axis out"=w856:u8, "connection ID"=w857:refnum<k5>)  [unwired: 4 in, 1 out]
                        n377 = call "ControlTargetRange.vi"("Set"=FALSE, "error in"=w855, "axis in"=w856, "connection ID"=w857) -> ("error out"=w849:errorcluster, "Target Range out"=w850:dbl)  [unwired: 4 in, 2 out]
                        n378 = local write "Target Range 3"(w850) -> ()
                      }
                      event "auto Reset 3": Value Change {
                        n379 = event-data() -> ()  [unwired: 1 in, 1 out]
                        n380 = call "controlAutoReset.vi"("Set"=TRUE, "auto reset in"="auto Reset 3", "axis in"=w863, "connection ID"=w864) -> ("error out"=w860:errorcluster, "axis out"=w866:u8, "connection ID"=w867:refnum<k5>)  [unwired: 4 in, 1 out]
                        n381 = call "controlAutoReset.vi"("Set"=FALSE, "error in"=w860, "axis in"=w866, "connection ID"=w867) -> ("error out"=w859:errorcluster, "auto reset out"=w861:bool)  [unwired: 4 in, 2 out]
                        n382 = local write "auto Reset 3"(w861) -> ()
                      }
                      event "Reference Auto Update 3": Value Change {
                        n383 = event-data() -> ()  [unwired: 1 in, 1 out]
                        n384 = call "controlReferenceAutoUpdate.vi"("Set"=TRUE, "ref auto up in"="Reference Auto Update 3", "axis in"=w871, "connection ID"=w873) -> ("error out"=w874:errorcluster, "axis out"=w875:u8, "connection ID"=w876:refnum<k5>)  [unwired: 4 in, 1 out]
                        n385 = call "controlReferenceAutoUpdate.vi"("Set"=FALSE, "error in"=w874, "axis in"=w875, "connection ID"=w876) -> ("error out"=w869:errorcluster, "ref auto up out"=w870:bool)  [unwired: 4 in, 2 out]
                        n386 = local write "Reference Auto Update 3"(w870) -> ()
                      }
                      event Timeout {
                        n387 = event-data() -> ()  [unwired: 1 in, 1 out]
                        n388 = call "getPosition.vi"("axis in"=w899, "connection ID"=w900) -> ("error out"=w898:errorcluster, "position out"=→"Position 3":dbl, "axis out"=w914:u8, "connection ID"=w915:refnum<k5>)  [unwired: 6 in]
                        n389 = call "getReferencePosition.vi"("error in"=w898, "axis in"=w914, "connection ID"=w915) -> ("error out"=w897:errorcluster, "Reference position out"=→"Reference 3":dbl, "axis out"=w912:u8, "connection ID"=w913:refnum<k5>)  [unwired: 5 in]
                        n390 = call "getStatusConnected.vi"("error in"=w897, "axis in"=w912, "connection ID"=w913) -> ("error out"=w896:errorcluster, "Status Connected out"=→"Connected 3":bool, "axis out"=w910:u8, "connection ID"=w911:refnum<k5>)  [unwired: 5 in]
                        n391 = call "getStatusMoving.vi"("error in"=w896, "axis in"=w910, "connection ID"=w911) -> ("error out"=w895:errorcluster, "status moving out"=→"MoveSignal 3":bool, "axis out"=w908:u8, "connection ID"=w909:refnum<k5>)  [unwired: 5 in]
                        n392 = call "getStatusReference.vi"("error in"=w895, "axis in"=w908, "connection ID"=w909) -> ("error out"=w894:errorcluster, "status reference out"=→"ReferenceSignal 3":bool, "axis out"=w906:u8, "connection ID"=w907:refnum<k5>)  [unwired: 5 in]
                        n393 = call "getStatusEotBkwd.vi"("error in"=w894, "axis in"=w906, "connection ID"=w907) -> ("error out"=w893:errorcluster, "Get Stus EOT BKWD out"=→"EotLeftDetected3":bool, "axis out"=w904:u8, "connection ID"=w905:refnum<k5>)  [unwired: 5 in]
                        n394 = call "getStatusEotFwd.vi"("error in"=w893, "axis in"=w904, "connection ID"=w905) -> ("error out"=w901:errorcluster, "Status EOT FWD out"=→"EotrightDetected3":bool, "axis out"=w902:u8, "connection ID"=w903:refnum<k5>)  [unwired: 5 in]
                        n395 = call "getStatusTargetRange.vi"("error in"=w901, "axis in"=w902, "connection ID"=w903) -> ("error out"=w882:errorcluster, "Status Target Range out"=→"in target range3":bool, "axis out"=w883:u8, "connection ID"=w884:refnum<k5>)  [unwired: 5 in]
                        n396 = call "ControlMove.vi"("Set"=FALSE, "error in"=w882, "axis in"=w883, "connection ID"=w884) -> ("error out"=w881:errorcluster, "controll move out"=w879:bool)  [unwired: 4 in, 2 out]
                        n397 = local write "move out 3"(w879) -> ()
                        n398 = local write "Move 3"(w879) -> ()
                      }
                    }
                    n399 = Unbundle(w729) -> ("code"=w728:i32, "source"=w730:string)  [unwired: 1 out]
                    n400 = Not Equal To 0?(x=w728) -> (x != 0?=w727:bool)
                    n401 = case shown="False" w727 {
                      selector: w727 -> [_ w733]
                      tunnel: w730 -> [_ w734]
                      frame False {
                      }
                      frame True {
                        "Error Message 3" <- w734
                        "Error 3" <- w733
                      }
                    }
                  }
                }
              }
              frame "Interface" {
                n402 = stacked-sequence {
                  tunnel: w916 -> [w917 w1042 w1167]
                  frame #0 {
                    w923 = u8 0 items=["1", "2", "3"] ("axis in")
                    n403 = event shown="[0] Timeout" {
                      selector: _ -> [_ _ _ _ _ _ _ _ _ _ _]
                      dyn-events: _ -> [_ _ _ _ _ _ _ _ _ _ _]
                      timeout: 10 -> [_ _ _ _ _ _ _ _ _ _ _]
                      tunnel: w923 -> [w933 w957 w968 w977 w987 w995 w1004 w1017 w1025 w1035 _]
                      tunnel: [_ w952 w963 w971 w984 w991 w1000 w1012 w1020 w1032 _] -> w920
                      tunnel: w917 -> [w934 w959 w969 w979 w989 w999 w1009 w1019 w1029 w1039 _]
                      event Timeout {
                        n404 = event-data() -> ()  [unwired: 1 in, 1 out]
                        n405 = call "controlRealtimeInputMode.vi"("Set"=FALSE ("set"), "axis in"=w933, "connection ID"=w934) -> ("error out"=w926:errorcluster, "RT Mode out"=w931:i32, "axis out"=w927:u8, "connection ID"=w928:refnum<k5>)  [unwired: 5 in]
                        n406 = local write "Mode Input 1"(w931) -> ()
                        n407 = Equal?(x=w931, y=15) -> (x = y?=w937:bool)
                        n408 = call "controlRealtimeInputLoopMode.vi"("Set"=FALSE ("set"), "error in"=w926, "axis in"=w927, "connection ID"=w928) -> ("RT Loop out"=w930:i32)  [unwired: 4 in, 3 out]
                        n409 = local write "Loop Mode 1"(w930) -> ()
                        n410 = Equal?(x=w930, y=0) -> (x = y?=w935:bool)
                        n411 = case shown="True" w937 {
                          tunnel: w935 -> [w939 _]
                          frame False {
                            n412 = case shown="True" w939 {
                              frame False {
                                w940 = T1."Enabled" ("Disabled")
                                n413 = property on="RT in move 1" class="Bool (strict)"("DisabledEnum"=w940) -> ()  [unwired: 2 in, 2 out]
                                n414 = property on="RT in move Signal 1" class="Bool (strict)"("DisabledEnum"=w940) -> ()  [unwired: 2 in, 2 out]
                                n415 = property on="Loop Mode 1" class="Ring (strict)"("DisabledEnum"=w940) -> ()  [unwired: 2 in, 2 out]
                                n416 = property on="Steps per pulse 1" class="DigNum (strict)"("DisabledEnum"=T1."Disabled and Grayed Out" ("Disabled")) -> ()  [unwired: 2 in, 2 out]
                                n417 = property on="Change per pulse 1" class="DigNum (strict)"("DisabledEnum"=w940) -> ()  [unwired: 2 in, 2 out]
                              }
                              frame True {
                                w943 = T1."Enabled" ("Disabled")
                                w942 = T1."Disabled and Grayed Out" ("Disabled")
                                n418 = property on="RT in move 1" class="Bool (strict)"("DisabledEnum"=w942) -> ()  [unwired: 2 in, 2 out]
                                n419 = property on="RT in move Signal 1" class="Bool (strict)"("DisabledEnum"=w942) -> ()  [unwired: 2 in, 2 out]
                                n420 = property on="Loop Mode 1" class="Ring (strict)"("DisabledEnum"=w943) -> ()  [unwired: 2 in, 2 out]
                                n421 = property on="Steps per pulse 1" class="DigNum (strict)"("DisabledEnum"=w943) -> ()  [unwired: 2 in, 2 out]
                                n422 = property on="Change per pulse 1" class="DigNum (strict)"("DisabledEnum"=w942) -> ()  [unwired: 2 in, 2 out]
                              }
                            }
                          }
                          frame True {
                            w944 = T1."Disabled and Grayed Out" ("Disabled")
                            n423 = property on="RT in move 1" class="Bool (strict)"("DisabledEnum"=w944) -> ()  [unwired: 2 in, 2 out]
                            n424 = property on="RT in move Signal 1" class="Bool (strict)"("DisabledEnum"=w944) -> ()  [unwired: 2 in, 2 out]
                            n425 = property on="Loop Mode 1" class="Ring (strict)"("DisabledEnum"=w944) -> ()  [unwired: 2 in, 2 out]
                            n426 = property on="Steps per pulse 1" class="DigNum (strict)"("DisabledEnum"=w944) -> ()  [unwired: 2 in, 2 out]
                            n427 = property on="Change per pulse 1" class="DigNum (strict)"("DisabledEnum"=w944) -> ()  [unwired: 2 in, 2 out]
                          }
                        }
                      }
                      event "Mode Input 1": Value Change {
                        n428 = event-data() -> ()  [unwired: 1 in, 1 out]
                        n429 = call "controlRealtimeInputMode.vi"("Set"=TRUE, "RT Mode in"="Mode Input 1", "axis in"=w957, "connection ID"=w959) -> ("error out"=w953:errorcluster, "axis out"=w956:u8, "connection ID"=w958:refnum<k5>)  [unwired: 4 in, 1 out]
                        n430 = call "controlRealtimeInputMode.vi"("Set"=FALSE, "error in"=w953, "axis in"=w956, "connection ID"=w958) -> ("error out"=w946:errorcluster, "RT Mode out"=w948:i32, "axis out"=w950:u8, "connection ID"=w951:refnum<k5>)  [unwired: 4 in]
                        n431 = local write "Mode Input 1"(w948) -> ()
                        n432 = call "controlRealtimeInputLoopMode.vi"("Set"=FALSE, "error in"=w946, "axis in"=w950, "connection ID"=w951) -> ("error out"=w952:errorcluster, "RT Loop out"=w947:i32)  [unwired: 4 in, 2 out]
                        n433 = local write "Loop Mode 1"(w947) -> ()
                      }
                      event "Loop Mode 1": Value Change {
                        n434 = event-data() -> ()  [unwired: 1 in, 1 out]
                        n435 = call "controlRealtimeInputLoopMode.vi"("Set"=TRUE, "RT Loop in"="Loop Mode 1", "axis in"=w968, "connection ID"=w969) -> ("error out"=w964:errorcluster, "axis out"=w965:u8, "connection ID"=w966:refnum<k5>)  [unwired: 4 in, 1 out]
                        n436 = call "controlRealtimeInputLoopMode.vi"("Set"=FALSE, "error in"=w964, "axis in"=w965, "connection ID"=w966) -> ("error out"=w963:errorcluster, "RT Loop out"=w961:i32)  [unwired: 4 in, 2 out]
                        n437 = local write "Loop Mode 1"(w961) -> ()
                      }
                      event "Steps per pulse 1": Value Change {
                        n438 = event-data() -> ()  [unwired: 1 in, 1 out]
                        n439 = call "controlRealtimeInputStepsPerPulse.vi"("Set"=TRUE, "Steps in"="Steps per pulse 1", "axis in"=w977, "connection ID"=w979) -> ("error out"=w972:errorcluster, "axis out"=w973:u8, "connection ID"=w978:refnum<k5>)  [unwired: 4 in, 1 out]
                        n440 = call "controlRealtimeInputStepsPerPulse.vi"("Set"=FALSE, "error in"=w972, "axis in"=w973, "connection ID"=w978) -> ("error out"=w971:errorcluster, "Steps out"=w970:i32)  [unwired: 4 in, 2 out]
                        n441 = local write "Steps per pulse 1"(w970) -> ()
                      }
                      event "Change per pulse 1": Value Change {
                        n442 = event-data() -> ()  [unwired: 1 in, 1 out]
                        n443 = call "controlRealTimeInChangePerPulse.vi"("Set"=TRUE, "Change in"="Change per pulse 1", "axis in"=w987, "connection ID"=w989) -> ("error out"=w985:errorcluster, "axis out"=w983:u8, "connection ID"=w988:refnum<k5>)  [unwired: 4 in, 1 out]
                        n444 = call "controlRealTimeInChangePerPulse.vi"("Set"=FALSE, "error in"=w985, "axis in"=w983, "connection ID"=w988) -> ("error out"=w984:errorcluster, "Change out"=w982:i32)  [unwired: 4 in, 2 out]
                        n445 = local write "Change per pulse 1"(w982) -> ()
                      }
                      event "RT in move 1": Value Change {
                        n446 = event-data() -> ()  [unwired: 1 in, 1 out]
                        n447 = call "controlRealtimeInputMove.vi"("Set"=TRUE, "move in"="RT in move 1", "axis in"=w995, "connection ID"=w999) -> ("error out"=w992:errorcluster, "axis out"=w993:u8, "connection ID"=w998:refnum<k5>)  [unwired: 4 in, 1 out]
                        n448 = call "controlRealtimeInputMove.vi"("Set"=FALSE, "error in"=w992, "axis in"=w993, "connection ID"=w998) -> ("error out"=w991:errorcluster, "move out"=→"RT in move Signal 1":bool)  [unwired: 4 in, 2 out]
                      }
                      event "AquadB in res 1": Value Change {
                        n449 = event-data() -> ()  [unwired: 1 in, 1 out]
                        n450 = call "controlAQuadBInResolution.vi"("Set"=TRUE, "Resolution in"="AquadB in res 1", "axis in"=w1004, "connection ID"=w1009) -> ("error out"=w1001:errorcluster, "axis out"=w1007:u8, "connection ID"=w1008:refnum<k5>)  [unwired: 3 in, 1 out]
                        n451 = call "controlAQuadBInResolution.vi"("Set"=FALSE, "error in"=w1001, "axis in"=w1007, "connection ID"=w1008) -> ("error out"=w1000:errorcluster, "Resolution out"=w1002:i32)  [unwired: 3 in, 2 out]
                        n452 = local write "AquadB in res 1"(w1002) -> ()
                      }
                      event "AquadB out 1": Value Change {
                        n453 = event-data() -> ()  [unwired: 1 in, 1 out]
                        n454 = call "controlAQuadBOut.vi"("Set"=TRUE, "ABout in"="AquadB out 1", "axis in"=w1017, "connection ID"=w1019) -> ("error out"=w1013:errorcluster, "axis out"=w1010:u8, "connection ID"=w1018:refnum<k5>)  [unwired: 4 in, 1 out]
                        n455 = call "controlAQuadBOut.vi"("Set"=FALSE, "error in"=w1013, "axis in"=w1010, "connection ID"=w1018) -> ("error out"=w1012:errorcluster, "ABout out"=w1011:bool)  [unwired: 4 in, 2 out]
                        n456 = local write "AquadB out 1"(w1011) -> ()
                      }
                      event "AqaudB clock 1": Value Change {
                        n457 = event-data() -> ()  [unwired: 1 in, 1 out]
                        n458 = call "controlAQuadBOutClock.vi"("Set"=TRUE, "clock in"="AqaudB clock 1", "axis in"=w1025, "connection ID"=w1029) -> ("error out"=w1022:errorcluster, "axis out"=w1024:u8, "connection ID"=w1028:refnum<k5>)  [unwired: 4 in, 1 out]
                        n459 = call "controlAQuadBOutClock.vi"("Set"=FALSE, "error in"=w1022, "axis in"=w1024, "connection ID"=w1028) -> ("error out"=w1020:errorcluster, "clock out"=w1021:i32)  [unwired: 4 in, 2 out]
                        n460 = local write "AqaudB clock 1"(w1021) -> ()
                      }
                      event "AquadB Resolution 1": Value Change {
                        n461 = event-data() -> ()  [unwired: 1 in, 1 out]
                        n462 = call "controlAQuadBOutResolution.vi"("Set"=TRUE, "ABoutRes in"="AquadB Resolution 1", "axis in"=w1035, "connection ID"=w1039) -> ("error out"=w1033:errorcluster, "axis out"=w1034:u8, "connection ID"=w1038:refnum<k5>)  [unwired: 4 in, 1 out]
                        n463 = call "controlAQuadBOutResolution.vi"("Set"=FALSE, "error in"=w1033, "axis in"=w1034, "connection ID"=w1038) -> ("error out"=w1032:errorcluster, "ABoutRes out"=w1030:i32)  [unwired: 4 in, 2 out]
                        n464 = local write "AquadB Resolution 1"(w1030) -> ()
                      }
                      event "Reset Error 4": Value Change {
                        n465 = event-data() -> ()  [unwired: 1 in, 1 out]
                        n466 = local write "Error Message 4"("" ("Error Message")) -> ()
                        n467 = local write "Error 4"(FALSE ("Error 4")) -> ()
                      }
                    }
                    n468 = Unbundle(w920) -> ("code"=w918:i32, "source"=w919:string)  [unwired: 1 out]
                    n469 = Not Equal To 0?(x=w918) -> (x != 0?=w921:bool)
                    n470 = case shown="True" w921 {
                      selector: w921 -> [_ w924]
                      tunnel: w919 -> [_ w925]
                      frame False {
                      }
                      frame True {
                        "Error Message 4" <- w925
                        "Error 4" <- w924
                      }
                    }
                  }
                  frame #1 {
                    w1048 = u8 1 items=["1", "2", "3"] ("axis in")
                    n471 = event shown="[4] \"Change per pulse 2\": Value Change" {
                      selector: _ -> [_ _ _ _ _ _ _ _ _ _ _]
                      dyn-events: _ -> [_ _ _ _ _ _ _ _ _ _ _]
                      timeout: 1 -> [_ _ _ _ _ _ _ _ _ _ _]
                      tunnel: w1048 -> [w1057 w1076 w1087 w1098 w1110 w1117 w1127 w1138 w1147 w1157 _]
                      tunnel: [_ w1070 w1089 w1096 w1105 w1118 w1128 w1139 w1148 w1158 _] -> w1043
                      tunnel: w1042 -> [w1058 w1077 w1090 w1099 w1111 w1119 w1129 w1140 w1149 w1159 _]
                      event Timeout {
                        n472 = event-data() -> ()  [unwired: 1 in, 1 out]
                        n473 = call "controlRealtimeInputMode.vi"("Set"=FALSE ("set"), "axis in"=w1057, "connection ID"=w1058) -> ("error out"=w1051:errorcluster, "RT Mode out"=w1056:i32, "axis out"=w1052:u8, "connection ID"=w1053:refnum<k5>)  [unwired: 5 in]
                        n474 = local write "Mode Input 2"(w1056) -> ()
                        n475 = Equal?(x=w1056, y=15) -> (x = y?=w1062:bool)
                        n476 = call "controlRealtimeInputLoopMode.vi"("Set"=FALSE ("set"), "error in"=w1051, "axis in"=w1052, "connection ID"=w1053) -> ("RT Loop out"=w1055:i32)  [unwired: 4 in, 3 out]
                        n477 = local write "Loop Mode 2"(w1055) -> ()
                        n478 = Equal?(x=w1055, y=0) -> (x = y?=w1060:bool)
                        n479 = case shown="False" w1062 {
                          tunnel: w1060 -> [w1064 _]
                          frame False {
                            n480 = case shown="False" w1064 {
                              frame False {
                                w1065 = T1."Enabled" ("Disabled")
                                n481 = property on="RT in move 2" class="Bool (strict)"("DisabledEnum"=w1065) -> ()  [unwired: 2 in, 2 out]
                                n482 = property on="RT in move Signal 2" class="Bool (strict)"("DisabledEnum"=w1065) -> ()  [unwired: 2 in, 2 out]
                                n483 = property on="Loop Mode 2" class="Ring (strict)"("DisabledEnum"=w1065) -> ()  [unwired: 2 in, 2 out]
                                n484 = property on="Steps per pulse 2" class="DigNum (strict)"("DisabledEnum"=T1."Disabled and Grayed Out" ("Disabled")) -> ()  [unwired: 2 in, 2 out]
                                n485 = property on="Change per pulse 2" class="DigNum (strict)"("DisabledEnum"=w1065) -> ()  [unwired: 2 in, 2 out]
                              }
                              frame True {
                                w1068 = T1."Enabled" ("Disabled")
                                w1067 = T1."Disabled and Grayed Out" ("Disabled")
                                n486 = property on="RT in move 2" class="Bool (strict)"("DisabledEnum"=w1067) -> ()  [unwired: 2 in, 2 out]
                                n487 = property on="RT in move Signal 2" class="Bool (strict)"("DisabledEnum"=w1067) -> ()  [unwired: 2 in, 2 out]
                                n488 = property on="Loop Mode 2" class="Ring (strict)"("DisabledEnum"=w1068) -> ()  [unwired: 2 in, 2 out]
                                n489 = property on="Steps per pulse 2" class="DigNum (strict)"("DisabledEnum"=w1068) -> ()  [unwired: 2 in, 2 out]
                                n490 = property on="Change per pulse 2" class="DigNum (strict)"("DisabledEnum"=w1067) -> ()  [unwired: 2 in, 2 out]
                              }
                            }
                          }
                          frame True {
                            w1069 = T1."Disabled and Grayed Out" ("Disabled")
                            n491 = property on="RT in move 2" class="Bool (strict)"("DisabledEnum"=w1069) -> ()  [unwired: 2 in, 2 out]
                            n492 = property on="RT in move Signal 2" class="Bool (strict)"("DisabledEnum"=w1069) -> ()  [unwired: 2 in, 2 out]
                            n493 = property on="Loop Mode 2" class="Ring (strict)"("DisabledEnum"=w1069) -> ()  [unwired: 2 in, 2 out]
                            n494 = property on="Steps per pulse 2" class="DigNum (strict)"("DisabledEnum"=w1069) -> ()  [unwired: 2 in, 2 out]
                            n495 = property on="Change per pulse 2" class="DigNum (strict)"("DisabledEnum"=w1069) -> ()  [unwired: 2 in, 2 out]
                          }
                        }
                      }
                      event "Mode Input 2": Value Change {
                        n496 = event-data() -> ()  [unwired: 1 in, 1 out]
                        n497 = call "controlRealtimeInputMode.vi"("Set"=TRUE, "RT Mode in"="Mode Input 2", "axis in"=w1076, "connection ID"=w1077) -> ("error out"=w1072:errorcluster, "axis out"=w1082:u8, "connection ID"=w1084:refnum<k5>)  [unwired: 4 in, 1 out]
                        n498 = call "controlRealtimeInputMode.vi"("Set"=FALSE, "error in"=w1072, "axis in"=w1082, "connection ID"=w1084) -> ("error out"=w1071:errorcluster, "RT Mode out"=w1074:i32, "axis out"=w1081:u8, "connection ID"=w1083:refnum<k5>)  [unwired: 4 in]
                        n499 = local write "Mode Input 2"(w1074) -> ()
                        n500 = call "controlRealtimeInputLoopMode.vi"("Set"=FALSE, "error in"=w1071, "axis in"=w1081, "connection ID"=w1083) -> ("error out"=w1070:errorcluster, "RT Loop out"=w1073:i32)  [unwired: 4 in, 2 out]
                        n501 = local write "Loop Mode 2"(w1073) -> ()
                      }
                      event "Loop Mode 2": Value Change {
                        n502 = event-data() -> ()  [unwired: 1 in, 1 out]
                        n503 = call "controlRealtimeInputLoopMode.vi"("Set"=TRUE, "RT Loop in"="Loop Mode 2", "axis in"=w1087, "connection ID"=w1090) -> ("error out"=w1091:errorcluster, "axis out"=w1092:u8, "connection ID"=w1093:refnum<k5>)  [unwired: 4 in, 1 out]
                        n504 = call "controlRealtimeInputLoopMode.vi"("Set"=FALSE, "error in"=w1091, "axis in"=w1092, "connection ID"=w1093) -> ("error out"=w1089:errorcluster, "RT Loop out"=w1086:i32)  [unwired: 4 in, 2 out]
                        n505 = local write "Loop Mode 2"(w1086) -> ()
                      }
                      event "Steps per pulse 2": Value Change {
                        n506 = event-data() -> ()  [unwired: 1 in, 1 out]
                        n507 = call "controlRealtimeInputStepsPerPulse.vi"("Set"=TRUE, "Steps in"="Steps per pulse 2", "axis in"=w1098, "connection ID"=w1099) -> ("error out"=w1100:errorcluster, "axis out"=w1101:u8, "connection ID"=w1104:refnum<k5>)  [unwired: 4 in, 1 out]
                        n508 = call "controlRealtimeInputStepsPerPulse.vi"("Set"=FALSE, "error in"=w1100, "axis in"=w1101, "connection ID"=w1104) -> ("error out"=w1096:errorcluster, "Steps out"=w1095:i32)  [unwired: 4 in, 2 out]
                        n509 = local write "Steps per pulse 2"(w1095) -> ()
                      }
                      event "Change per pulse 2": Value Change {
                        n510 = event-data() -> ()  [unwired: 1 in, 1 out]
                        n511 = call "controlRealTimeInChangePerPulse.vi"("Set"=TRUE, "Change in"="Change per pulse 2", "axis in"=w1110, "connection ID"=w1111) -> ("error out"=w1113:errorcluster, "axis out"=w1112:u8, "connection ID"=w1114:refnum<k5>)  [unwired: 4 in, 1 out]
                        n512 = call "controlRealTimeInChangePerPulse.vi"("Set"=FALSE, "error in"=w1113, "axis in"=w1112, "connection ID"=w1114) -> ("error out"=w1105:errorcluster, "Change out"=w1106:i32)  [unwired: 4 in, 2 out]
                        n513 = local write "Change per pulse 2"(w1106) -> ()
                      }
                      event "RT in move 2": Value Change {
                        n514 = event-data() -> ()  [unwired: 1 in, 1 out]
                        n515 = call "controlRealtimeInputMove.vi"("Set"=TRUE, "move in"="RT in move 2", "axis in"=w1117, "connection ID"=w1119) -> ("error out"=w1120:errorcluster, "axis out"=w1121:u8, "connection ID"=w1124:refnum<k5>)  [unwired: 4 in, 1 out]
                        n516 = call "controlRealtimeInputMove.vi"("Set"=FALSE, "error in"=w1120, "axis in"=w1121, "connection ID"=w1124) -> ("error out"=w1118:errorcluster, "move out"=→"RT in move Signal 2":bool)  [unwired: 4 in, 2 out]
                      }
                      event "AquadB in res 2": Value Change {
                        n517 = event-data() -> ()  [unwired: 1 in, 1 out]
                        n518 = call "controlAQuadBInResolution.vi"("Set"=TRUE, "Resolution in"="AquadB in res 2", "axis in"=w1127, "connection ID"=w1129) -> ("error out"=w1130:errorcluster, "axis out"=w1133:u8, "connection ID"=w1134:refnum<k5>)  [unwired: 3 in, 1 out]
                        n519 = call "controlAQuadBInResolution.vi"("Set"=FALSE, "error in"=w1130, "axis in"=w1133, "connection ID"=w1134) -> ("error out"=w1128:errorcluster, "Resolution out"=w1125:i32)  [unwired: 3 in, 2 out]
                        n520 = local write "AquadB in res 2"(w1125) -> ()
                      }
                      event "AquadB out 2": Value Change {
                        n521 = event-data() -> ()  [unwired: 1 in, 1 out]
                        n522 = call "controlAQuadBOut.vi"("Set"=TRUE, "ABout in"="AquadB out 2", "axis in"=w1138, "connection ID"=w1140) -> ("error out"=w1141:errorcluster, "axis out"=w1137:u8, "connection ID"=w1144:refnum<k5>)  [unwired: 4 in, 1 out]
                        n523 = call "controlAQuadBOut.vi"("Set"=FALSE, "error in"=w1141, "axis in"=w1137, "connection ID"=w1144) -> ("error out"=w1139:errorcluster, "ABout out"=w1135:bool)  [unwired: 4 in, 2 out]
                        n524 = local write "AquadB out 2"(w1135) -> ()
                      }
                      event "AqaudB clock 2": Value Change {
                        n525 = event-data() -> ()  [unwired: 1 in, 1 out]
                        n526 = call "controlAQuadBOutClock.vi"("Set"=TRUE, "clock in"="AqaudB clock 2", "axis in"=w1147, "connection ID"=w1149) -> ("error out"=w1150:errorcluster, "axis out"=w1151:u8, "connection ID"=w1154:refnum<k5>)  [unwired: 4 in, 1 out]
                        n527 = call "controlAQuadBOutClock.vi"("Set"=FALSE, "error in"=w1150, "axis in"=w1151, "connection ID"=w1154) -> ("error out"=w1148:errorcluster, "clock out"=w1145:i32)  [unwired: 4 in, 2 out]
                        n528 = local write "AqaudB clock 2"(w1145) -> ()
                      }
                      event "AquadB Resolution 2": Value Change {
                        n529 = event-data() -> ()  [unwired: 1 in, 1 out]
                        n530 = call "controlAQuadBOutResolution.vi"("Set"=TRUE, "ABoutRes in"="AquadB Resolution 2", "axis in"=w1157, "connection ID"=w1159) -> ("error out"=w1160:errorcluster, "axis out"=w1161:u8, "connection ID"=w1164:refnum<k5>)  [unwired: 4 in, 1 out]
                        n531 = call "controlAQuadBOutResolution.vi"("Set"=FALSE, "error in"=w1160, "axis in"=w1161, "connection ID"=w1164) -> ("error out"=w1158:errorcluster, "ABoutRes out"=w1155:i32)  [unwired: 4 in, 2 out]
                        n532 = local write "AquadB Resolution 2"(w1155) -> ()
                      }
                      event "Reset Error 5": Value Change {
                        n533 = event-data() -> ()  [unwired: 1 in, 1 out]
                        n534 = local write "Error 5"(FALSE ("Error 5")) -> ()
                        n535 = local write "Error Message 5"("" ("Error Message")) -> ()
                      }
                    }
                    n536 = Unbundle(w1043) -> ("code"=w1045:i32, "source"=w1044:string)  [unwired: 1 out]
                    n537 = Not Equal To 0?(x=w1045) -> (x != 0?=w1046:bool)
                    n538 = case shown="True" w1046 {
                      selector: w1046 -> [_ w1049]
                      tunnel: w1044 -> [_ w1050]
                      frame False {
                      }
                      frame True {
                        "Error Message 5" <- w1050
                        "Error 5" <- w1049
                      }
                    }
                  }
                  frame #2 {
                    w1172 = u8 2 items=["1", "2", "3"] ("axis in")
                    n539 = event shown="[8] \"AquadB out 3\": Value Change" {
                      selector: _ -> [_ _ _ _ _ _ _ _ _ _ _ _]
                      dyn-events: _ -> [_ _ _ _ _ _ _ _ _ _ _ _]
                      timeout: 1 -> [_ _ _ _ _ _ _ _ _ _ _ _]
                      tunnel: w1172 -> [w1182 w1197 w1214 w1223 w1232 w1242 w1253 _ w1271 w1281 w1291 _]
                      tunnel: [_ w1199 w1211 w1220 w1233 w1243 w1252 w1261 w1268 w1278 w1288 _] -> w1168
                      tunnel: w1167 -> [w1183 w1202 w1215 w1224 w1234 w1244 w1254 w1267 w1272 w1282 w1292 _]
                      event Timeout {
                        n540 = event-data() -> ()  [unwired: 1 in, 1 out]
                        n541 = call "controlRealtimeInputMode.vi"("Set"=FALSE ("set"), "axis in"=w1182, "connection ID"=w1183) -> ("error out"=w1176:errorcluster, "RT Mode out"=w1181:i32, "axis out"=w1177:u8, "connection ID"=w1178:refnum<k5>)  [unwired: 5 in]
                        n542 = local write "Mode Input 3"(w1181) -> ()
                        n543 = Equal?(x=w1181, y=15) -> (x = y?=w1187:bool)
                        n544 = call "controlRealtimeInputLoopMode.vi"("Set"=FALSE ("set"), "error in"=w1176, "axis in"=w1177, "connection ID"=w1178) -> ("RT Loop out"=w1180:i32)  [unwired: 4 in, 3 out]
                        n545 = local write "Loop Mode 3"(w1180) -> ()
                        n546 = Equal?(x=w1180, y=0) -> (x = y?=w1185:bool)
                        n547 = case shown="False" w1187 {
                          tunnel: w1185 -> [w1189 _]
                          frame False {
                            n548 = case shown="True" w1189 {
                              frame False {
                                w1190 = T1."Enabled" ("Disabled")
                                n549 = property on="RT in move 3" class="Bool (strict)"("DisabledEnum"=w1190) -> ()  [unwired: 2 in, 2 out]
                                n550 = property on="RT in move Signal 3" class="Bool (strict)"("DisabledEnum"=w1190) -> ()  [unwired: 2 in, 2 out]
                                n551 = property on="Loop Mode 3" class="Ring (strict)"("DisabledEnum"=w1190) -> ()  [unwired: 2 in, 2 out]
                                n552 = property on="Steps per pulse 3" class="DigNum (strict)"("DisabledEnum"=T1."Disabled and Grayed Out" ("Disabled")) -> ()  [unwired: 2 in, 2 out]
                                n553 = property on="Change per pulse 3" class="DigNum (strict)"("DisabledEnum"=w1190) -> ()  [unwired: 2 in, 2 out]
                              }
                              frame True {
                                w1193 = T1."Enabled" ("Disabled")
                                w1192 = T1."Disabled and Grayed Out" ("Disabled")
                                n554 = property on="RT in move 3" class="Bool (strict)"("DisabledEnum"=w1192) -> ()  [unwired: 2 in, 2 out]
                                n555 = property on="RT in move Signal 3" class="Bool (strict)"("DisabledEnum"=w1192) -> ()  [unwired: 2 in, 2 out]
                                n556 = property on="Loop Mode 3" class="Ring (strict)"("DisabledEnum"=w1193) -> ()  [unwired: 2 in, 2 out]
                                n557 = property on="Steps per pulse 3" class="DigNum (strict)"("DisabledEnum"=w1193) -> ()  [unwired: 2 in, 2 out]
                                n558 = property on="Change per pulse 3" class="DigNum (strict)"("DisabledEnum"=w1192) -> ()  [unwired: 2 in, 2 out]
                              }
                            }
                          }
                          frame True {
                            w1194 = T1."Disabled and Grayed Out" ("Disabled")
                            n559 = property on="RT in move 3" class="Bool (strict)"("DisabledEnum"=w1194) -> ()  [unwired: 2 in, 2 out]
                            n560 = property on="RT in move Signal 3" class="Bool (strict)"("DisabledEnum"=w1194) -> ()  [unwired: 2 in, 2 out]
                            n561 = property on="Loop Mode 3" class="Ring (strict)"("DisabledEnum"=w1194) -> ()  [unwired: 2 in, 2 out]
                            n562 = property on="Steps per pulse 3" class="DigNum (strict)"("DisabledEnum"=w1194) -> ()  [unwired: 2 in, 2 out]
                            n563 = property on="Change per pulse 3" class="DigNum (strict)"("DisabledEnum"=w1194) -> ()  [unwired: 2 in, 2 out]
                          }
                        }
                      }
                      event "Mode Input 3": Value Change {
                        n564 = event-data() -> ()  [unwired: 1 in, 1 out]
                        n565 = call "controlRealtimeInputMode.vi"("Set"=TRUE, "RT Mode in"="Mode Input 3", "axis in"=w1197, "connection ID"=w1202) -> ("error out"=w1201:errorcluster, "axis out"=w1207:u8, "connection ID"=w1209:refnum<k5>)  [unwired: 4 in, 1 out]
                        n566 = call "controlRealtimeInputMode.vi"("Set"=FALSE, "error in"=w1201, "axis in"=w1207, "connection ID"=w1209) -> ("error out"=w1200:errorcluster, "RT Mode out"=w1196:i32, "axis out"=w1206:u8, "connection ID"=w1208:refnum<k5>)  [unwired: 4 in]
                        n567 = local write "Mode Input 3"(w1196) -> ()
                        n568 = call "controlRealtimeInputLoopMode.vi"("Set"=FALSE, "error in"=w1200, "axis in"=w1206, "connection ID"=w1208) -> ("error out"=w1199:errorcluster, "RT Loop out"=w1195:i32)  [unwired: 4 in, 2 out]
                        n569 = local write "Loop Mode 3"(w1195) -> ()
                      }
                      event "Loop Mode 3": Value Change {
                        n570 = event-data() -> ()  [unwired: 1 in, 1 out]
                        n571 = call "controlRealtimeInputLoopMode.vi"("Set"=TRUE, "RT Loop in"="Loop Mode 3", "axis in"=w1214, "connection ID"=w1215) -> ("error out"=w1216:errorcluster, "axis out"=w1217:u8, "connection ID"=w1218:refnum<k5>)  [unwired: 4 in, 1 out]
                        n572 = call "controlRealtimeInputLoopMode.vi"("Set"=FALSE, "error in"=w1216, "axis in"=w1217, "connection ID"=w1218) -> ("error out"=w1211:errorcluster, "RT Loop out"=w1212:i32)  [unwired: 4 in, 2 out]
                        n573 = local write "Loop Mode 3"(w1212) -> ()
                      }
                      event "Steps per pulse 3": Value Change {
                        n574 = event-data() -> ()  [unwired: 1 in, 1 out]
                        n575 = call "controlRealtimeInputStepsPerPulse.vi"("Set"=TRUE, "Steps in"="Steps per pulse 3", "axis in"=w1223, "connection ID"=w1224) -> ("error out"=w1225:errorcluster, "axis out"=w1226:u8, "connection ID"=w1229:refnum<k5>)  [unwired: 4 in, 1 out]
                        n576 = call "controlRealtimeInputStepsPerPulse.vi"("Set"=FALSE, "error in"=w1225, "axis in"=w1226, "connection ID"=w1229) -> ("error out"=w1220:errorcluster, "Steps out"=w1221:i32)  [unwired: 4 in, 2 out]
                        n577 = local write "Steps per pulse 3"(w1221) -> ()
                      }
                      event "Change per pulse 3": Value Change {
                        n578 = event-data() -> ()  [unwired: 1 in, 1 out]
                        n579 = call "controlRealTimeInChangePerPulse.vi"("Set"=TRUE, "Change in"="Change per pulse 3", "axis in"=w1232, "connection ID"=w1234) -> ("error out"=w1238:errorcluster, "axis out"=w1237:u8, "connection ID"=w1239:refnum<k5>)  [unwired: 4 in, 1 out]
                        n580 = call "controlRealTimeInChangePerPulse.vi"("Set"=FALSE, "error in"=w1238, "axis in"=w1237, "connection ID"=w1239) -> ("error out"=w1233:errorcluster, "Change out"=w1230:i32)  [unwired: 4 in, 2 out]
                        n581 = local write "Change per pulse 3"(w1230) -> ()
                      }
                      event "RT in move 3": Value Change {
                        n582 = event-data() -> ()  [unwired: 1 in, 1 out]
                        n583 = call "controlRealtimeInputMove.vi"("Set"=TRUE, "move in"="RT in move 3", "axis in"=w1242, "connection ID"=w1244) -> ("error out"=w1245:errorcluster, "axis out"=w1246:u8, "connection ID"=w1249:refnum<k5>)  [unwired: 4 in, 1 out]
                        n584 = call "controlRealtimeInputMove.vi"("Set"=FALSE, "error in"=w1245, "axis in"=w1246, "connection ID"=w1249) -> ("error out"=w1243:errorcluster, "move out"=→"RT in move Signal 3":bool)  [unwired: 4 in, 2 out]
                      }
                      event "AquadB in res 3": Value Change {
                        n585 = event-data() -> ()  [unwired: 1 in, 1 out]
                        n586 = call "controlAQuadBInResolution.vi"("Set"=TRUE, "Resolution in"="AquadB in res 3", "axis in"=w1253, "connection ID"=w1254) -> ("error out"=w1255:errorcluster, "axis out"=w1258:u8, "connection ID"=w1259:refnum<k5>)  [unwired: 3 in, 1 out]
                        n587 = call "controlAQuadBInResolution.vi"("Set"=FALSE, "error in"=w1255, "axis in"=w1258, "connection ID"=w1259) -> ("error out"=w1252:errorcluster, "Resolution out"=w1250:i32)  [unwired: 3 in, 2 out]
                        n588 = local write "AquadB in res 3"(w1250) -> ()
                      }
                      event "Output Mode": Value Change {
                        n589 = event-data() -> ()  [unwired: 1 in, 1 out]
                        n590 = call "controlRtOutSignalMode.vi"("Set"=TRUE, "RT out Mode in"="Output Mode", "connection ID"=w1267) -> ("error out"=w1262:errorcluster, "connection ID"=w1266:refnum<k5>)  [unwired: 6 in, 1 out]
                        n591 = call "controlRtOutSignalMode.vi"("Set"=FALSE, "error in"=w1262, "connection ID"=w1266) -> ("error out"=w1261:errorcluster, "RT out Mode out"=w1260:i32)  [unwired: 6 in, 1 out]
                        n592 = local write "Output Mode"(w1260) -> ()
                      }
                      event "AquadB out 3": Value Change {
                        n593 = event-data() -> ()  [unwired: 1 in, 1 out]
                        n594 = call "controlAQuadBOut.vi"("Set"=TRUE, "ABout in"="AquadB out 3", "axis in"=w1271, "connection ID"=w1272) -> ("error out"=w1274:errorcluster, "axis out"=w1273:u8, "connection ID"=w1277:refnum<k5>)  [unwired: 4 in, 1 out]
                        n595 = call "controlAQuadBOut.vi"("Set"=FALSE, "error in"=w1274, "axis in"=w1273, "connection ID"=w1277) -> ("error out"=w1268:errorcluster, "ABout out"=w1269:bool)  [unwired: 4 in, 2 out]
                        n596 = local write "AquadB out 3"(w1269) -> ()
                      }
                      event "AqaudB clock 3": Value Change {
                        n597 = event-data() -> ()  [unwired: 1 in, 1 out]
                        n598 = call "controlAQuadBOutClock.vi"("Set"=TRUE, "clock in"="AqaudB clock 3", "axis in"=w1281, "connection ID"=w1282) -> ("error out"=w1283:errorcluster, "axis out"=w1284:u8, "connection ID"=w1287:refnum<k5>)  [unwired: 4 in, 1 out]
                        n599 = call "controlAQuadBOutClock.vi"("Set"=FALSE, "error in"=w1283, "axis in"=w1284, "connection ID"=w1287) -> ("error out"=w1278:errorcluster, "clock out"=w1279:i32)  [unwired: 4 in, 2 out]
                        n600 = local write "AqaudB clock 3"(w1279) -> ()
                      }
                      event "AquadB Resolution 3": Value Change {
                        n601 = event-data() -> ()  [unwired: 1 in, 1 out]
                        n602 = call "controlAQuadBOutResolution.vi"("Set"=TRUE, "ABoutRes in"="AquadB Resolution 3", "axis in"=w1291, "connection ID"=w1292) -> ("error out"=w1293:errorcluster, "axis out"=w1294:u8, "connection ID"=w1297:refnum<k5>)  [unwired: 4 in, 1 out]
                        n603 = call "controlAQuadBOutResolution.vi"("Set"=FALSE, "error in"=w1293, "axis in"=w1294, "connection ID"=w1297) -> ("error out"=w1288:errorcluster, "ABoutRes out"=w1289:i32)  [unwired: 4 in, 2 out]
                        n604 = local write "AquadB Resolution 3"(w1289) -> ()
                      }
                      event "Reset Error 6": Value Change {
                        n605 = event-data() -> ()  [unwired: 1 in, 1 out]
                        n606 = local write "Error 6"(FALSE ("Error 6")) -> ()
                        n607 = local write "Error Message 6"("" ("Error Message")) -> ()
                      }
                    }
                    n608 = Unbundle(w1168) -> ("code"=w1170:i32, "source"=w1171:string)  [unwired: 1 out]
                    n609 = Not Equal To 0?(x=w1170) -> (x != 0?=w1169:bool)
                    n610 = case shown="True" w1169 {
                      selector: w1169 -> [_ w1174]
                      tunnel: w1171 -> [_ w1175]
                      frame False {
                      }
                      frame True {
                        "Error Message 6" <- w1175
                        "Error 6" <- w1174
                      }
                    }
                  }
                }
              }
              frame "About" {
                n611 = event shown="[7] \"Reset Error 8\": Value Change" {
                  selector: _ -> [_ _ _ _ _ _ _ _]
                  dyn-events: _ -> [_ _ _ _ _ _ _ _]
                  timeout: 10 -> [_ _ _ _ _ _ _ _]
                  tunnel: w1304 -> [w1314 w1317 w1320 w1322 w1325 w1327 w1329 _]
                  tunnel: [w1310 w1316 w1318 w1321 w1323 w1326 w1328 _] -> w1300
                  event Timeout {
                    n612 = event-data() -> ()  [unwired: 1 in, 1 out]
                    n613 = call "getDeviceName.vi"("connection ID in"=w1314) -> ("error out"=w1311:errorcluster, "Device Name out"=→"Name":string, "connection ID out"=w1312:refnum<k5>)  [unwired: 8 in]
                    n614 = call "getLockStatus.vi"("error in"=w1311, "connection ID in"=w1312) -> ("error out"=w1310:errorcluster, "locked"=→"locked":bool, "authorized"=→"authorized":bool)  [unwired: 6 in, 1 out]
                  }
                  event "name": Value Change {
                    n615 = event-data() -> ()  [unwired: 1 in, 1 out]
                    n616 = call "setDeviceName.vi"("device name in"="name", "connection ID"=w1317) -> ("error out"=w1316:errorcluster)  [unwired: 8 in, 1 out]
                  }
                  event "Lock password": Value Change {
                    n617 = event-data() -> ()  [unwired: 1 in, 1 out]
                    n618 = call "lock.vi"("password"="Lock password", "connection ID"=w1320) -> ("error out"=w1318:errorcluster)  [unwired: 8 in, 1 out]
                  }
                  event "Unlock": Value Change {
                    n619 = event-data() -> ()  [unwired: 1 in, 1 out]
                    n620 = call "unlock.vi"("connection ID"=w1322) -> ("error out"=w1321:errorcluster)  [unwired: 9 in, 1 out]
                  }
                  event "Access Password": Value Change {
                    n621 = event-data() -> ()  [unwired: 1 in, 1 out]
                    n622 = call "grantAccess.vi"("password"="Access Password", "connection ID"=w1325) -> ("error out"=w1323:errorcluster)  [unwired: 8 in, 1 out]
                  }
                  event "Reboot": Value Change {
                    n623 = event-data() -> ()  [unwired: 1 in, 1 out]
                    n624 = call "rebootSystem.vi"("connection ID"=w1327) -> ("error out"=w1326:errorcluster)  [unwired: 9 in, 1 out]
                  }
                  event "Factory Reset": Value Change {
                    n625 = event-data() -> ()  [unwired: 1 in, 1 out]
                    n626 = call "factoryReset.vi"("connection ID"=w1329) -> ("error out"=w1328:errorcluster)  [unwired: 9 in, 1 out]
                  }
                  event "Reset Error 8": Value Change {
                    n627 = event-data() -> ()  [unwired: 1 in, 1 out]
                    n628 = local write "Error 7"(FALSE ("Error 7")) -> ()
                    n629 = local write "Error Message 7"("" ("Error Message 9")) -> ()
                  }
                }
                n630 = Unbundle(w1300) -> ("code"=w1303:i32, "source"=w1301:string)  [unwired: 1 out]
                n631 = Not Equal To 0?(x=w1303) -> (x != 0?=w1302:bool)
                n632 = case shown="True" w1302 {
                  selector: w1302 -> [_ w1307]
                  tunnel: w1301 -> [_ w1306]
                  frame False {
                  }
                  frame True {
                    "Error Message 7" <- w1306
                    "Error 7" <- w1307
                  }
                }
              }
            }
          }
        }
        frame #2 {
          # "Exit / Disconnect"
          n633 = local write "stop"(FALSE ("stop")) -> ()
          n634 = call "close.vi"("connection ID"=w1332) -> ()  [unwired: 6 in, 1 out]
        }
      }
    }
    frame True {
    }
  }
